vi "player tansition data for all.vi"() -> ()   [LabVIEW 2013]
panel:
  in  "DU opp ALL":string[](array[string])=["0 3 0 1 0 -3 0 -3 3 0\r\n", "1 -4\r\n", "2 0 2 0 -1 0 -3\r\n", "0 4\r\n", "0 -1 2 -1 0 2 0 3 0 1 -4 1 0 -4 4 -4\r\n", "0 -1 0 -4 0 -2 0\r\n", "1 -1 1 0 -4\r\n", "-1 0 -4 0 1 0\r\n", "0 3\r\n", "-1 1 0 -4 1 0 -4 0 -1 2 0\r\n", "1 0 -1 0 2\r\n", "0 -1 -4 1 0 -3 3\r\n", "2 -1 0\r\n", "0 4 0 2 0 -3 0 1 -1 0 1 -4 4 -4 4 -4 0 3\r\n", "0 -4 4 -4 0 -1 2 0 3 -3 0 -3 3 0 -4 1 0 -3 0 3 -2\r\n", "0 3 0\r\n", "0 4 0 1 0 -4 4\r\n", "0 -1 0 4 0\r\n", "1 -1 0 4 0 2 -2 0 -4 1 -4 4 -3 0 -4 0 -3 3 0 -4 1 -1 2 -1 0 4\r\n", "0 3 0 4 -4 4 -4 1 -4 1 -4 4 -4 1 -4 0 -3 3\r\n", "", "0\r\n", "0 4 -4 0 -4 0 4 -4 0\r\n", "1 -4\r\n", "0 4\r\n", "0 1 -4 1 -4 0 -4 4 -4 0\r\n", "-2 2 0 -3 3 -3 0 3 0\r\n", "1 0 4 0\r\n", "0 3 0 1 0\r\n", "0 4 -4 0 -4 1 -4 0\r\n", "0\r\n", "0 -4 4 -4 0 -3 3 -2 0 2\r\n", "0 3 0 1 0 -4 4 0 -3 3 0 -4 0\r\n", "0 1 0 3 -2 3\r\n", "0 2 -2 3 -3 0 -3 3 -2 2 0 -4 4 -4 1 0 4 0 2 -2 0 4 0 4 0 2 -2 2\r\n", "0 -3 3 0 -2\r\n", "1 0 -2 0 4 0 1 0 -2 2 -2\r\n", "-2 0 3 0\r\n", "-4 0 -2 0 3 -3 0 -2 2 -2 0 -4 0 3 -2 0\r\n", "0 -3 4 0 1 0 -2\r\n", "-2\r\n", "-4 0\r\n", "-2 0 -3 4 -3 4 -4\r\n", "0 1 -4 0 -2 2 -2 0 -4 0 -3 3 -2 3 0 1 0\r\n", "0 3\r\n", "0 2 0 3 0 1 0 -2 2 -2 3 0\r\n", "-1 0 -1 1 0 4 -4 4 -4\r\n", "0 -3 4 -3 -2 2 -2 3 -2 2 -2 0\r\n", "2 0 -3 3\r\n", "0 3 0 -1 0\r\n", "0 3\r\n", "0 3 0 3\r\n", "-4 0 -4 1 -4\r\n", "2 -2 0 3 -3 0 1 0 -1 0 4 -3 0 2 -2 0\r\n", "0 1 0 4 -4 4 0\r\n", "0 1 0 -3 3 -3 0\r\n", "0 -3 4 0 -4 1 0 -2\r\n", "0 3 0 -2\r\n", "2 0 -3 3 -2 2 0 -2 0 -3 4 -3\r\n", "0 1 0 3 0\r\n", "0 3 0 -2\r\n", "-4 0 3 0 2 -1 0 3 0\r\n", "2 0 4 0 -2 2\r\n", "0 -3 4 -3 0 -2 2 -2 0 4\r\n", "0 3 -2 0 -3 4 0 3 0 1 -1 0 -1 0\r\n", "0 -3 4 -3 0\r\n", "2 0 3 -3 0 -4 0 -2\r\n", "-1 0 3 -3 0 1 0 4\r\n", "0 1 0\r\n", "0 -1 0 -1 1 -1 0\r\n", "0 -3 3 -3 0 1 -4 0 -1 0\r\n", "2 0 3 -2 0 -2 3 -2 0\r\n", "0 1 0\r\n", "2 0\r\n", "0 1 -4 0 -4 0 -3 4 -4 0 2 0 2\r\n", "0 3 -2 2 0 -4 0 -3 0 1 -4 4 0 2 0 -3 3 -3 0 -2 2 0\r\n", "0 2 0 3 -3 0 3 -3 0 1 0 4 -3 0 2 0 -2 0 4 -4 1 -1\r\n", "-4 1 0\r\n", "0 2 0\r\n", "0 1 0 -4 0 -4 0 -1 0\r\n", "0 4 -4 0 -4 4 -3 0 2 0 -1 1 -1 0 3\r\n", "0 2 0 -4\r\n", "0 3 -2 0 -2 0 -2 3 -2 2 -2 3\r\n", "0\r\n", "0 -3 4 0\r\n", "0 2 0\r\n", "0 -3 4 -3 0 -2 2\r\n", "0\r\n", "0 2 0 1 0 -3 4\r\n", "2 0 -4 1 0 3 0 -4 1 -1 0 4 -4 1 0 2 -2\r\n", "1\r\n", "2 0 -1 0 -1\r\n", "1 0 4 -4 0 2 0 -1 0 -1 0 4 -4 0 2 0 3 -2 3 0 -1 1 0 4\r\n", "0 1 0 -2 0 -1 1 -4 4 0 -4 0\r\n", "0 -1 0 -1 0\r\n", "2 0 -1 1 0 4 -4 1 0 1 0 -3 0 -2 0 -4 0 4 0 1 0\r\n", "0 4 -4 1 -4 1 -4 0 -1 0 -1 0 -1 1 0 -4 4 0 -1 0\r\n", "0 3 -2 0 3 0 2 0 2 0 -4 1 0 -3 0 1 0 4 -4 0 3 -3 0 1 0 -1 0 -1 -4 4 0 2\r\n", "1 -4 1 -1 0 -4 1\r\n", "2 -1 0 -4 1 0\r\n", "1\r\n", "2 0 1 0 -4 1 -4 4\r\n", "0 2 0 -2 2 -1 0 4 -4 0 -4 4\r\n", "1 0\r\n", "2 0 -4 4 0 2 -1 0 -4 4 0 1 -1 0 4 0 2\r\n", "0 4 -4 1 -4 0 -4 1 -4 4 -4 0 1 -1\r\n", "0 -1 1 0 -4 0 -1 0 3 -2\r\n", "1 -4 1 0 1 -4 4 -4 1 0 1 -4 1 0 4 0 4 -4 0 4 -4 1 0 4\r\n", "2 0\r\n", "1 0 1 0 -3 0 -3 3 -2 2 -1 0 -1 0 -1 0 -4 1 0 2 -2 2 0 4 -3 0 4 -4 1 0 4 0 -1 2 0 -3 0 3 0 1\r\n", "2 0 2 0 -4 4 -4 0 -4 4 -3 0 2\r\n", "0 3 0 2 -1\r\n", "0 4 0 -2 0 3\r\n", "0 4 -4 1 0 -4 0 4 -4 0 2 0 -1 1 -1 0 -1\r\n", "1 0 4 -4 1 0 4 -4 0\r\n", "2 -1 0 -1 0 4\r\n", "1 -4 1 0 4 0 2 0 2 0 -3 0\r\n", "2 -1 0 -3 0\r\n", "0 -1 1 0 1 -4 4 -4 0 -1 0 -3 3 0 1 0\r\n", "0 2 0 3 0\r\n", "1 0 1 -4 1 0\r\n", "2 0 3 0 3\r\n", "0 3 0\r\n", "0 2 0 3 0 3 0 3 -2 0 1 -4 1 -4 4 -4 1 -4 4 -4 4 -4 1 -4 0 -2 0 1 0 -4 4 -4 0\r\n", "0 4 0 -2 0 1 -4 4 -4 1\r\n", "0 4 -4 1 -4 1 0 1 -4 1 -4 1 -4 0 2 0 3 0 2 0 -3 3 0 3 -2 0 -1 1\r\n", "1 0 1 -4 1 0 -1 0 -4 0 -1 0 4 0 4\r\n", "0 1 0 1 0 1 -4 1 -4 4 0 -1 0 3 0 -1 0 4 0 2 0 2 0 4 -4 4\r\n", "0 2 0 1 0 -4 1 0 4\r\n", "2 0 -1 0 2 0 4 0 -2 0 3 0 2 0 2 -2 2\r\n", "0\r\n", "0 2 0 -2 0 -1 1 -1 0 -4 1 -4 1 -4 1 0 -4 4 0 -4 0\r\n", "1 0 -1 0 1 -4 1\r\n", "2 -1\r\n", "0 1 0 3 0 1 0 4 0 4 -4 1\r\n", "0 4 0 2 0 1 0 1 0\r\n", "-4 1 0 -4 0 -2 0 2 -1 0 4 -4 1 0 4 -4 0 2 0\r\n", "0 -3 3 0 1 0 1 0 -4 4 -4 0 1 0 4 -4\r\n", "2 0 1 0 1 0 2 0 3 -2 3\r\n", "0 4 0 2 0 -2 2 0 -4 4 -4 0 3 0 4 0 2 -1 0 4 -4 0 -4 4 0 2 0 -2 3 -2 2 -1 0 -4 4 -4 0 2 0 -3 0 -3 3 0 4 -4 0 2 -1 1 -4 4 0 2\r\n", "1 0 -4 1 -4 0 -4 4 0 -1 0 -4 1 0 1 -4 1 -4 1 -1 0 4 -4 0 3 0 -1\r\n", "0 -3 3\r\n", "0 1 0 -3 4 -3 0 2 -2 0 -2 0 -3 4 -3 0 -2 2 -2 0 -3 4 0 2 0\r\n", "-4 0 -4 4\r\n", "0 4\r\n", "0 2 0\r\n", "-4 0\r\n", "0 -3 0\r\n", "-2 2 0 -3 3 0 3 -3 0 -2 2 -2 3 -3 3 -2 0 -3 4 0 4\r\n", "0 -3 3 0 2 0 -4 1 0\r\n", "-4 1 -4 4 0 1 -1 0 3\r\n", "0 -3 4 0 -3 3 -3 0 -2 0 -4 0 -2 0 -3 3 0 1 0 -4 4 0 -3 3 0 3\r\n", "0 4 0 -4 0 -1 0 1 -4 4 -4 0\r\n", "0 1 0 -3 4 0 2\r\n", "0 2 0 3 -3 -4 1 -4 4 -3 4 0 -4 0 -3 4 -3 0 -2 2 0 -4 0 3 -2 3 -2 0 -3 3 0\r\n", "-4 1 0 -4 0 3 -2 0 -3 4 0 2 0 3 -3 0 1 -4 0 2 -2 0 -2 0 -3 3 0 3\r\n", "0 -2 2 -2 0 -2 2 0 3\r\n", "0 -3 3 0 3\r\n", "0 2 0 4 0 2 -2 0 -3 4 0 1 -4 0 -2 2 0 -4 1 0\r\n", "0 -3 3 -3 0 1 0 3\r\n", "0\r\n", "0\r\n", "0 4 0 -2 0 -3 4 -3 0\r\n", "0 1 -4 0 -4 0 2 -2 3 0 2 0 1\r\n", "0 3 0\r\n", "0 -3 3 -3 0 3\r\n", "0 3 0 4 -4 0 -3 3 -3 0 2 0 2 0 4\r\n", "0 4\r\n", "0 2 0 -4 0 1 0 1 -4 0 4 0\r\n", "0 2 -2 0 3\r\n", "-4\r\n", "2 0 1 -4 0 4\r\n", "0 4 0\r\n", "2\r\n", "0 1 -4 0 4 -3 0 -4\r\n", "0 2 0 3\r\n", "0 2 0 -3 3\r\n", "0 2 0 -2 2 -2 0 -3 4 -4 1 0 -3 4 0\r\n", "0 -4 0 -4 1 0 2 0 2 0 3 -3 0 -4 1 0 3 -2 2 0 -3 4 -3 0 3 0 3\r\n"]
  in  "CL opp ALL":string[](array[string])=["0 3 -2 0 -2 0 -2 0 -2 2 -2 0 3 -3 0 2 0 -3 4 -3 0\r\n", "0\r\n", "0 3 -3 0\r\n", "0 2 -2 0 3 -3 0 1 -4 -1 1 0 -4 0 3 0\r\n", "-4 1 0 2 -1 0 3 -3 0 -4 0 2 0 3 0 -4 1\r\n", "0 2 0\r\n", "0 3 -2 0 3 -3 0 3 0 2 0 3 0 3 0 -2 2 -2 0 -2 3\r\n", "-4 1 0 -2 3 0 -1 0 3 0\r\n", "0 1 -4 0 -4 0 3 0 2 -2 0 4 -4 1 0 3 -3 0 -2 3 0 -4 0 2 0 -4 0\r\n", "0 -4 4 -3 0 3\r\n", "0 3 -2 3\r\n", "0\r\n", "0 -3 3 -3 0 2 0 3 0 -2 2\r\n", "-4 1 0 3 0 -3 -2 3 0 1 -4 0 3 -3 0 1 0 -2 0 2 0\r\n", "-1 0 -2 3 -2 0\r\n", "0 3 0 3 -3 0 -4 0 -3 3 -3 0 -4 0 4 -3 0 1 -4\r\n", "-4 0 -2 0 3 -3 0 -3 3 0 -4 0 2 0 -4 0 2 -2 0 -3\r\n", "0 3 0 -3 4 0 2 0 3 -3 0 -4\r\n", "0 3 -2 0 4 0 -2 0 3 -3 0 3 0 3 -3 0 -2 0 4 -3 0\r\n", "0 4 0\r\n", "0 2 0 -4 0 -4 0 3 -2 0 -3 3 0 2 -2 3 -3 0 -4 1 0 -4 0 -2 0 4 0 -2 0 -2 0 1 0 4 0 -2 2 -2 0 3\r\n", "0 4 0 -2 2 0 3 0 -4 1 -4 0\r\n", "-4 0 -4 0 -4 0 -3\r\n", "0 4 -4 1 -4\r\n", "-4 0 -2 3 -2 3 0 -4 4 -4 4 -4 0 4\r\n", "0 3 0 -2 0 1 0 4\r\n", "0 3 0 2 0\r\n", "0 3 0 -4 0 3 -3 0 -4 1 0 4\r\n", "0 4 -4 4 -4 0 -1 0\r\n", "-2 0 3 0 -4 0 -2 2 0 3 -3 0 -2 2 -2 -3 3 -3\r\n", "-4 0 -3 0 3 -2 0 3 -2 2 -1 0\r\n", "0 3 -3 0 1 -4 0\r\n", "0 2 0\r\n", "0\r\n", "-4 0 4 0 -4 0 -4 4 0 2 0 4 -3 0 2 -2 0 -2 3 0 -2 2 -2 0 -2 0 -2 3 -3 0 4 0 4 -4 1 0 -3 3 0 -4\r\n", "0 -2 3 0 -4 1 -4 0 -2 2 -2 0 -2 3 -3\r\n", "-4 0 -2 3 0 2 -2 3 0 3 -3 0 -3 3 -3 0 3 -3 4 0 2 0 4 0 -4 0\r\n", "0 3 0 3 0 -1 2 0 3 -3\r\n", "0 3 -3 0 2 0 3 -3 0 -3 3 -2 0 1 0 1 0\r\n", "-4 0 -3 3 -2 2 -2 0 3 -3 0 -2 2 0\r\n", "0 3 -3 0 -4 1 0 4 0 -3 3 -3 0 -4 1 -4 0\r\n", "0 2 0\r\n", "-4 0 4 -4 4 -4 0 4 0 2 0 3 0 3 -2 2 0\r\n", "0 3 -2 0 3 0 -2 2 0\r\n", "0\r\n", "0 3 -3 0 -4 0 -4 0 -2 0\r\n", "-4 0 -4 0 -3 3 0 3 -3 0 -4 1 0\r\n", "0 3 0 -3 4 -4 1 -4 0 -3 3 -3 0 -2 2 0 1 0 -2 0 -4 1\r\n", "0 2 -2 3 -3 0 4 -4 4 0 2 0 3 -3 0 -2 0 1 0\r\n", "0 3 -2 0 3 -3 0 1 -4 1 0\r\n", "-4 0 -4 0 3 0 3 0 3 0 2 0 -2 0 -2 0 -3 3 -3 0 1 0 3 -3 0 -2 0 4 0 -4 0 -2 3 0 -4 1 -4 1 0 4 0 -2 2 0 -4 0 3 0 -4\r\n", "0 3 0 3 0 -2 0 3 -3 0 3 0 2 0 -3 4 -4 1 0 3 -3 0 1 0\r\n", "0 2 0\r\n", "0 -1 0 4 0 -1 0 1 -4 4 -4 1 0 -4 1 -4 0 1 0 4 -4 0\r\n", "0 -2 0 2 0\r\n", "1 -1 0\r\n", "0\r\n", "-1 0 3 0 4\r\n", "0 2 0 4\r\n", "0 -1 0 -4 0 1 -4 1 0 -4 1 0 3 0\r\n", "1 -1 0 -4 0 -3 4 0 -1 0 3 -2 2 0 -3 0\r\n", "0 -1 0 2 0 3 0 2 0 4 0\r\n", "0 3 0 1 -1 0 -1 2 -1 0 1 -4 1 0 2 0 3 0 -4 0 2 0 1 0 2 0 -2 0 1\r\n", "2 0 -2 3 0 -1 0 -1 0 -1 0 3 0 2 0 4\r\n", "0 3 -2 0 1 0 -1 0\r\n", "0 -4 4 0 2 -1 0 1 0 1 0 3 0 4 0 -4 4 -4 0 -4 0 -1 2 -1 0 1 -4 1 0 -2 0\r\n", "0 3 0 3 -2 0 -4 0 -4 0 3 0 1 0 -2 3 0 -4 4 -4 0 2 0 3 0 -4 4 -4 0 2 0 4 -4 0\r\n", "1 -4 1 -4 4 -4 1 -4 1 -4 0 -3 3 0\r\n", "2 -1 0 4 -4\r\n", "1 0 3 0 2 0 -4 1 0 -2 0 -2 3 0 1 -4 1 0 3 -2 2 -1 0 -3 4\r\n", "0 3 -2 0 -1 0 3 0 -2 0 -4 4 0\r\n", "-1 0\r\n", "-1 0 -2 0\r\n", "1 -1 0 3 0 1 0 1\r\n", "2 0 2 0 -2 3 -2 0 -1 0 3 0 1 0 3 -2 -1 0 4 0 2 -1 1\r\n", "1 0 -2\r\n", "2 -1 0 -1 0 4 0\r\n", "0 3 0 1 -4 0 -1 0 3 -2 0 1 -4 1 0 1 0 3 0 -4 1 0 3 0\r\n", "-1 0 3 0 3 0\r\n", "1 -1 0 3 -2 0 -1 0 -1 0 3 -2 2 0 3 0 2 -2 0 3 0 -2 0\r\n", "0 3 0 4 -4 1 -4 1 0\r\n", "0 -1 0\r\n", "0 3 0 4 -4 0 3 0\r\n", "-1 0 3 -2 0 1 0\r\n", "0\r\n", "-1 0 4 0 2 0 -2 3\r\n", "2 -1 0 4 -4 0 -1 0\r\n", "-4 1 0 -1 0 -1 0 -4 4 -4 0 -1 0 -4\r\n", "2 -1 0 3 -2 0 1 -4 1 0 -2 0 1 -1 0 -2\r\n", "0 3 -2 2 0 3 -3 0 1 -4 1 0 -2 0 4 0 -4 1 -4 0 3 0 1 0 4 -4 0 -4 4 -4\r\n", "0 -1 0\r\n", "0 3 0 4 0\r\n", "0 2 0 -1 0 3 0 -1 0 -1 0 1 0 1\r\n", "0 -1 0 -2 -1 1 0 -3 0 3 0 2 -1 0 3 0 1 -4 4 0 4 -4 1 -4 4\r\n", "0 3 0 3 0 4 0 2 -2 0 4 -4 0 2 0 1 -4 4 -4 0 3 0\r\n", "0 -1 0 4\r\n", "1 0\r\n", "2 0 4 -4 0 1\r\n", "-4 1 -1 0 2 0 1 -4 0 -3 0 2 -2 0 4 0\r\n", "0 -1 0 3 0\r\n", "0 3 0 1 0 1\r\n", "0 -1 0 4 -4\r\n", "1 -1 0\r\n", "0 3 0 4\r\n", "2 0 -2 3 -2 0 4 0 -4 1 -4\r\n", "0 -1 0 3 -2\r\n", "0 -3 3 0\r\n", "0 3 0 -2 0 4 0 2 -2 0 4 0 4 -4 1 -4 0\r\n", "2 0 -3 3 0 -2 0 1\r\n", "0 3 0\r\n", "-4 0 2 0 3 -3 0 -3 4 0 -4 1\r\n", "-2 2 0 1 -1\r\n", "0 -1 0 4 -4 1 -4 1\r\n", "-4\r\n", "-2 2 0 3 0 -4 0 -3 3\r\n", "-4 1 0 4 -4 1 -4\r\n", "0 4 -4 0 4\r\n", "0 4 0 -4 0 1 -4 0 -4 4\r\n", "0 1 -4 0 -4 0 -2\r\n", "-2 2 0 -4 1 0 -4 0 4 0 3 0 -1 1 -1 1 0 -3 0 -2 2 0 -4 4 -4 0 2\r\n", "0 -3 3 -3 0\r\n", "-4 0 -1 2 0 -3 4 0 2 -2 0 3 -3 0 1 -4 0 -4 0 -4 0 -3 3 0 -3 4 0 2\r\n", "-2 0 3 0 -2 2 -2 0 -2 0\r\n", "-4 0 3 0 -4 1 0 -3 4\r\n", "-2 2 0 2 0 -2 0 -3 3 0 -4 1 0\r\n", "-4 0\r\n", "0 -3 3 0 2 0 -3 4 0 -2 0 1 -4 0\r\n", "0 2 0 3\r\n", "0 4 -4 1 -1 2 0 -3 0 1\r\n", "0 -2 0 -3 4 0 1 -4 0 -3 3 0 -4 0 4 0 2 -2 0 -2 0 -4\r\n", "0 3 -2 0 4 0 4 0 -1 0 -3 3 0 1 -4 0 -4 0 4 0 2 -2 0\r\n", "-2 3 -2 0 1 -4\r\n", "-4 0 -1 0 -3 3\r\n", "0 4\r\n", "0 3 0 -3 3 -3 0 -1 0 2 -2\r\n", "-2\r\n", "-4 0 -2 0 2 0 1 0 -4 0 4 0 2 0 -3 4 0 2 0 -2 0\r\n", "0 2\r\n", "-2 0\r\n", "-4 0 3 0 -4 1 -4 0 -4 4 -4 4\r\n", "0 1 -4 0 -3 3 0 1 -4 0\r\n", "-2\r\n", "-2 2 0 2 -1 0 4 0\r\n", "1 -4 1 0 -4 0 3 0 -1 0 -4 0 2 -2 0 4 0 2 0 4 -4 0 2 -2 0 1 0 -4 1 0 4 -4 0 1 -4 1 0 4 -4 0 2 0 4\r\n", "-2 2 0 -1 0\r\n", "0 -1 0 -1\r\n", "4 1 -1 0 4 -4 0 -1 0\r\n", "0 -2 2 0 -2 2 -2 0 4 -4 0 -1 0 -1\r\n", "0 -4 4 -4 -1 0 -1 0 1 -4 4\r\n", "-4 1 0 -1 0 -1 0 4 -4\r\n", "2 -1 0 1 0 4 -4 0 2\r\n", "0 1 0 4 -1 4 -4 1\r\n", "0 -1 0 4 0 -1 0 -1 0 2 -2\r\n", "-4 1 -4 1 0 1 0 -1 0 4 -4 0 2 0 3 -2 0 1 0 1 0 -1 2 -1 0\r\n", "-2 2 0 -1 2 -1 0 -3 3 0 -1 0 4 0 1 -4 0 -4 0 4 0 2 0\r\n", "1 0\r\n", "-2 2 -2 2 0 -3 0 1 -4 1 0 1 -4 1 -4 0 -3 3 0 4 0 1 -4 4 0\r\n", "1 -4 1 0 -4 1 0 -4 1\r\n", "0 -1 2 -2 2 0\r\n", "2 0\r\n", "-4 1 -4 1 0 -3 0 -1 0 1 -4 1 0 -1 1 -1 0 1 0 1 0 4 -1 4\r\n", "0 -4 0 1 -4 0 1 0 1 0 -3 3 0 2 -2 2\r\n", "-2 2 0 -1 0 -3 4 0\r\n", "0 1 -1 0 4 -4 1\r\n", "1 -4 1 0 4 -4 1\r\n", "0 4 -4 0 -1 0 -2 0 -1 0 -1 0 -3 3 0 -1 0 -1 0 -1 0 2 0 4 -4 1\r\n", "-2 2 0 2 -1 0 4 -4 0 -4 4 -4 -1 -4 1 0 -4 4 -4 0 2 -2 3 0 1 0\r\n", "1 -4 1 -4 0 -3 0 3\r\n", "0 -1 0 1\r\n", "0 -1 0 -1 0 -3 4 0 -4 0 -1 2 -1 0\r\n", "0 2 0\r\n", "1 -4 1 0\r\n", "2 0 4\r\n", "0 -1 0 -3 -1 -3 0 1 -4 0 -4 0 -3 0 1 -4 0 3 -2 -1 0 -4 1 0 -4 0 4 -4 0 2\r\n", "0 -1 0 1 0 -1 2 -1 0 -2 0 4\r\n", "0 -1 0 1\r\n", "0 1 -4 1 0 -1 0 -3 -1 -3\r\n", "0 -1 1\r\n", "0 -1 0 3 0 1 -4 1 0 4 0 -4 1 0\r\n"]
  in  "CJ opp left":string[](array[string])=["-2 2 -1 0 1 -4 0 3 -2\r\n", "1 -1 0 4 0 2 -2 3 0 1 -4 1 0 -3 4 0 3 0 4 0 4 0 -4 0\r\n", "-1 0 4 -4\r\n", "-1 0 -1 2 0 2 0\r\n", "-1 0 3 -2 0 2 -2 3 -2 2 -2 0 -3 4 0 1\r\n", "-2 2 -1 0 2 0 3 -1 3 -2 2 0 -2 2 -2 0 1 0 2 0\r\n", "1 -4 1 0 4 -4 0 2 0\r\n", "2 -2 0\r\n", "0 4 -4 -1 0 -1 1 -1 0 4 0 -2 3 -2 0\r\n", "-1 0 2 -1 0 4 -4 0 -4 0 4 0\r\n", "0 -3 0\r\n", "1 0 -1 2 -1 0 3 0 3 -2 3 -2 0 2\r\n", "2 0 2 0 -2 3 -2 2 -1 0 4 0 2\r\n", "-1 1 -4 1 0 1 0 -4 4 -4 0 3 -2 2 -1 0 3 0 -1 1\r\n", "2 0 -1 1 -1 0 3 -2 3 0 2 0 3 -2 0 -4 0 4 -4 0 4 0\r\n", "0 -1 0 3 0 2 -2\r\n", "1 -4 1 -1 0 2 0 3 -2 3 -2 3\r\n", "2 0\r\n", "-1 0 3 0 3\r\n", "1 -4 1 0 -4 4 -4 0\r\n", "-2 2 -1 0\r\n", "0 1 0 4 0 3 0 -2 0 3 0 4 0 2 -2 0\r\n", "0 3 -2 0 4 0 -2 2 -2 0 -2 0 4 0 -2 0 2\r\n", "2 0 1 -1 0\r\n", "1 0 -3 4 -3 0 -2 0 3 0\r\n", "0 3 -2 0 4 0 -3 3 0 3 -2 0\r\n", "2 0 3 0 1 0 3\r\n", "1 0 3 -3 0 4 -3 0\r\n", "-2 2 -2 0\r\n", "0 1 0 -3 4 0 3 -2 3 0 1 0 4 0 -1\r\n", "0 3\r\n", "-2 2 0 3 0 -2 0 2 0 -2 0 3 0 -4 0 -2\r\n", "0 3 0 -3 4\r\n", "0 3 -2 2 -2 3 -2 0\r\n", "-1 0 3 0 3\r\n", "2 0\r\n", "0 -3 0 1\r\n", "1 0 4 -4 1\r\n", "-2 2 0 4 0 -2 0 -2\r\n", "1 0 4 0 1 0 -3 3\r\n", "-2 2 0 3 -2\r\n", "1 0 -3 4 -3 0 3 0 3 0 -2 0 3 -2 0 1 -4 0 3 0 -2 0 3 -3 0\r\n", "-2 2 0 2 0 3\r\n", "0 3 -2 0 3 0 -4 1\r\n", "0 1 0 -4 4 0 -2 0 3 0 -4 0 4 0 -4 1 0 3 -2 3 0 -1 1 -1\r\n", "2 0 -3 4 -3 0 2 0\r\n", "0 3\r\n", "0 3\r\n", "-1 0 4\r\n", "0 3\r\n", "-2 3 0 1 -4 0 -2 2 -2 3 0 4\r\n", "2 -2 0 4 0 -4 1 -4 0 3 -2\r\n", "1 0 2\r\n", "0 3 0 2 -2 3 -3 0 1 0 -3 3 0 4 0 2 -2 2 -2 3 0\r\n", "2 0 -2 3 2\r\n", "0 1 0 4 -4 1 -1 2 -2 3 -3 0 -2\r\n", "0 -3 4 -3 0 2\r\n", "0 2 -2 3\r\n", "0 -4 0 -4 1 0 3 0 1 0 2 -2 0 -3 4 0 4 -3 0 3 -3 -2 0 -3 4 0 -4 0 3 0\r\n", "-2 2 -2 3 -3 0 -4 1\r\n", "0 -2 0 2 0 4 0\r\n", "0 -3 0 -4 0 -3 4 0 -2 3 -3\r\n", "2 0 -2 2 0 4 0 1 0 -2 3\r\n", "0 4 0 3 -2 3 0 -4 4 0 4 0 3 0 3\r\n", "2 0 -2 0 4 0 3 -2 2 -2 3 0 -2\r\n", "1 0 3 -3 0 3 0 3 -2 3 -2 3 0 3 0 -1 0 4 0 -4 1 0 3\r\n", "2 -2 0 -3 4 -3\r\n", "0 1 0 3 0 -2 2 -2\r\n", "1 0\r\n", "2 0 -2 3 -2 2 0\r\n", "1 0 -4 4 0 3 -2 3 -2 0 4 -3 0 -3 4 0 -4 1 -4 0 2 -2 0 3 -3 0 1 0 3 0 -2 3 0 4 0 -4 1 0 3 0 -3 4 0 2\r\n", "0 -3 4 -3 0 1 0\r\n", "0 3 0 4 0 -4 1 0 -2 0\r\n", "2 -2 0 -2 0 -4\r\n", "-1 0\r\n", "2 0 4\r\n", "1 0 3 0\r\n", "2 0 -4 4 0 1 0 3 -2 0 4 0 -4 0 3 0 -2 3\r\n", "0 2 -2 0 -4 0 -4 4 -3 0 -4 1 0 4 0 -3 3 0\r\n", "1 0 4 -3 0 2 -2 0 4 0 -3 4 -3 0 -4 0 -3 0 -4 1 0 -2 3 -2 0 1\r\n", "2 -2 3 0\r\n", "2 -1 0 4 0 1 0 3 -2\r\n", "0 3 0 -2 3 -2 0 -2 3 -2 2 -1 0 3 0\r\n", "1 0 1 0 4 -4 0 3 0 3 -2 0 4 0 3 -2\r\n", "0 3 -2 0 -1 1 0 2 -2 2 0 -3 4\r\n", "2 0 4\r\n", "0 -4 4 -4 0 1 -1 0 4\r\n", "-1 0 4 -4 0 -4 4 -4 0 2 0 -4 0 -3 3 -2 3 -2 0 -4\r\n", "2 0 -1 2 -1 0 1 -1 0 3 0 -2 0 3 0 -3 0 -3 0 -4 4 -4 1 -1 2 -1 1 0 3 0\r\n", "0 3\r\n", "1 0 -3 0 1 -4 0 2 0 -2 3 0 4 -4 0 -1 0 3 0 1\r\n", "0 -1 2 0 -3 4 0 -1 0 4 -4 4 -4 0 2 -1 1 0 -3 3 0\r\n", "0 3 -2 3 0 4 0 1 0 4 0 -4 4 -4 0 -4 4 -4 0 3\r\n", "2 0 3 0 1 0\r\n", "1 0 -4 1 -1 0 -2 -1 3 -2 2 -2 0 -3 0 1 -1\r\n", "2 0 3\r\n", "-4 1 -1 0 3 0 3 0 1\r\n", "0 4 0 -4 1 0 1 0 3 0 4 -4 0 -4 4 0\r\n", "2 0 -4 4 0 -1\r\n", "0 3 -2 2\r\n", "0 4 0 1 -4 4 -4 0 2 0 -3 4 0 4 -4 0 3 0 -1 1 -4 4 0 1\r\n", "0 1 -1 0 -4 0 4 0 1 0 4 0 2 0 -4 4 0 2 0 3 0 4 -4 0 3 0 4 0 -4 4\r\n", "1 0 -4 4 0 2 -1 0\r\n", "2 0 4 -4 1 -1 0 4 0 -2 2 0 4 -4 0 1 0 4 0 2\r\n", "0 4 0 3 -2 0 4\r\n", "0 3 0 -2 3 0 1 -4\r\n", "1 -4 1 0 -1 0 3 -2 2 0\r\n", "2 0 -1 0 3\r\n", "0 -1 0 2 0 -3 4 -4 0 3 0 1 -1 0 -4 4 -4 0 2 -1 1 0 3 0 4 -4 0 3 0 1 0 3 -2\r\n", "2 -1 0 3 0 4 -4 0 1 -4 1 -1 0 -4 4 0 -4 0 3 -2 0 4 -4 4 -4 0 2 -2 0 1 0 4 0 3 0 3 -2 3 -3 0 3 0 -3 0 1 -4\r\n", "1 -1 0 -2 3 -3 0 -4 0 -3 0 3 -2 0 3 -2 2\r\n", "0 4\r\n", "2 0 -2 3 0 2 -1 0 -3 0 -2 3\r\n", "1 0 3 0 3 0 -2 3 -2 0 -2 3 -2 0 3 0 1 -1 0 3 0 3 0 4 -4 0 1 -1 0 3 0 -3 0 -4 4 -4 0 3 0 -1 1 -4 1\r\n", "0 -1 2 0 3\r\n", "2 0 3 -2 0\r\n"]
  in  "CJ opp Right":string[](array[string])=["-2 0 3 0 -3 0 4 -4 0\r\n", "0 3\r\n", "0 4 -3 0 -4 1 0 4 -3 0\r\n", "0\r\n", "-2 0 3 -3 0 -4 1 -4 0 3 -3 4 -3 0 2 0 3\r\n", "0 3 0 1\r\n", "0 1 0 3\r\n", "0 3 -2 0 4\r\n", "0\r\n", "0 -3 4 0 2 -2 0 -3 0 3 -2 3 -3 4\r\n", "0 -3 4 -3 0\r\n", "-2 0 -2 2 0\r\n", "0 3 -2\r\n", "0 4 -3 0 3 -2 0 -3 4 -3 0 3 -2 2 -2 0 4 0\r\n", "2 0 1 -4 0 3 0 -4 4 0 -4 4 0 2 0 4 0 -3 4 -3 0 -4 0 4\r\n", "0 4\r\n", "-2 0 -2 0 3 0\r\n", "0 3 0 -2 3\r\n", "0 4 0 4 -4 0 2 0 -4 4 -3 0 -2 2 -2 0 4 -3 0 2 0 3 0\r\n", "0 4 -3 0 1 -1 0 3 0 -2 2 -2 0 -3 4 -3 0 4 -4 1 0\r\n", "", "0 -3\r\n", "2 0 3 0 1 0 -2 3\r\n", "0\r\n", "1 -1 0\r\n", "0 -2 3 0\r\n", "0 1 0 4 0 4 -4 4\r\n", "0 1 -1 0 3\r\n", "0 2 -2 3 -3 4\r\n", "-2 2 0 -2 3\r\n", "0 -1\r\n", "0 4 -4 4 0 3 0 -2 0 -4 0 1 -4\r\n", "-2 0 4 0 -3 3 0 -2 2 -2 0 -4 0 4 0\r\n", "0 -1 0 -4 4 -4 1 -4 0\r\n", "1 -4 1 0 2 0 -3 0 2 0 -2 0 1 0 1 -4 4 -4 1 0 3 -2 0 -4 4 -4\r\n", "0 1 -4 4 -4 1\r\n", "0 3 0 -3 3 0 1 0 1 -4 4\r\n", "0 1 -4 0 1 -4\r\n", "0 3 -2 0 1 -4 1 0 2 0 4 0 4 0 -1 2 -1 0\r\n", "1 0 -1 0 2 0 4 -4\r\n", "-4\r\n", "-1 0 4\r\n", "0 1 -1 0 1 -4 0\r\n", "-1 0 1 -4 0 3 0 2 0 4 0 -4 4 -4 0 -1 0 -4 0 -2 0 4\r\n", "0 4 0\r\n", "0 4 -4 0 2 -1 0 2 0 4 -4 1 -4 4 0 3\r\n", "0 4 0 2 0\r\n", "1 0 -1 1 0 -4 1 -4 1 0 -4\r\n", "0 3 -2 0 -4\r\n", "2 -1 0 -4 4 -4 0 2 0 4\r\n", "1 0\r\n", "-1 0 -1 1 0 -4\r\n", "0 3 0\r\n", "0 -4 4 -4 0 -4 0 4 0 2 0 1 -4 4\r\n", "-1 0 1 -4\r\n", "-1 0 2 -1 0 2\r\n", "1 -1 0 4 -4 1\r\n", "-1 0 1 -4 4 -4 0 -4 4\r\n", "0 3 0 3 0 1 -1 0 1\r\n", "-1 0 4 0 4 -4 1 0 -4 0\r\n", "1 0 4\r\n", "0 -1 0 2 -1 0 -2 3 -2 0 -4 4 -4\r\n", "0 3 0\r\n", "2 -1 0 1 -4 4 -4 0 2 0\r\n", "0 4 -4 1 0 1 0 1 -4 0 2 0 4 0 4 -4 1\r\n", "1 -1 0 3 0 3 0 1 0 4\r\n", "0 -4 0 -2 0 -4\r\n", "0 -4 4 -4 0 -2 0 2 0\r\n", "-1 0 4 -4 0\r\n", "1 0 -1 2 0 4\r\n", "0 2 0 -2 0\r\n", "0 1 -4 0 -4 0 3 -2 0 -4 0 -4 4 -4 1\r\n", "0 4 0 4 0 4 0 4 0 -2 3 0 3 0 4 0\r\n", "-4 -1\r\n", "-2 0 1 0 -4 4\r\n", "0 4\r\n", "-2 2 0 -1 -4 1 0 3 0\r\n", "-1 0 -1 2\r\n", "0 -1 1 0 4 0 3 -2 0 -2 3 -2 0 4 0 -2 2\r\n", "2 -1 0 4\r\n", "0 4 0 2 0 -2 0\r\n", "1 -1 0 3 0 -4 4 -4 0\r\n", "2 -1 0 3 -2 0 -3 0 3 0 -3 0\r\n", "0 4 0 4 -4 1 -1 0 -3 0 1 -4 1 0 4 0 -4 0 -4 4 -4 1\r\n", "0 -4 1 0 -4 4\r\n", "0 4 0 -2 2 -2 2 -2 2\r\n", "-2 2 -1 0 4 0 2 0 4 0 2 -2 0 4\r\n", "1 0 -1 0 -1 0 1 -1\r\n", "-2 2 -2 3\r\n", "1 0 -1 0 -1 2 0 2 -2 0 -4 0\r\n", "-2 2 0 3 -2 2\r\n", "0\r\n", "1 -1 0 3\r\n", "0 4 0\r\n", "-2 0 1 -4 0 -3 0\r\n", "1 0 -1 2 -1 1 -4\r\n", "0 4\r\n", "-2 0 -1 1\r\n", "0 3 0 3 0 3 -2\r\n", "-4 0 -4 4\r\n", "0 4 0 -4 0 -4\r\n", "-2 2 0 4 -4 0 2 -2\r\n", "-2 2 -2 0 -1\r\n", "0 4 -3 0\r\n", "0 1 0 -1 1\r\n", "-4 0\r\n", "-2 0 3 0 1 0 3 -2 0 -1 0 4 0 3 0 -3 3 -3\r\n", "0 4 0 -2 0 1 0 -4 4 -3 0 1 0 4 0 -4 1 0 3 -3 0\r\n", "0 -1 2\r\n", "2 0 -3 4 0\r\n", "-4 0 -3 3 -3 0 -3 3 0 -2 3 0\r\n", "0 -1 1 -4 4 -3 0 3 0\r\n", "0 -1 2 0 3 0 1 -4 4 0 2 0\r\n", "2 -2 0 -4 0 -4 4 0 -4\r\n", "1 -1 2 -1\r\n", "2 0 -2 0 4 0 2 0 3 0 -2 0 -4\r\n", "1 -1 0 -1\r\n", "0 1 -4 1\r\n", "0 4 0 -1 1 -1 0\r\n", "0 3\r\n", "-2 0\r\n", "1 -4 0 -2 0 4 0 -4 0 4 -3 0 1 -4 0 1\r\n", "0 -3 3 -2 0 3 0 -2 2\r\n", "1 0\r\n", "2\r\n", "0 -4\r\n", "0 4 0 -4 0 -3 3 -3 0 -2 0 -2 0 4 0 -1 1 0 3 0 -4 1 -4 0 4\r\n", "2 0 -1 1\r\n", "0 2 0 4 0 4 -4 0 -1 2\r\n", "0 3 -2 0 3 -2\r\n", "1 0 -3 3 0 -4\r\n", "0 -3 3 0 -1 0\r\n", "2 -2 0 1\r\n", "-4 1 -4 1 -4 0\r\n", "0 4 0 2 0 -4 1 2 -1 0 4 0 1 0 4 -4 4 0 -4 4 0\r\n", "-2 0 3 0 -2 0\r\n"]
  in  "CJ opp ALL":string[](array[string])=["-2 0 3 0 -3 0 4 -4 0\r\n", "0 3\r\n", "0 4 -3 0 -4 1 0 4 -3 0\r\n", "0\r\n", "-2 0 3 -3 0 -4 1 -4 0 3 -3 4 -3 0 2 0 3\r\n", "0 3 0 1\r\n", "0 1 0 3\r\n", "0 3 -2 0 4\r\n", "0\r\n", "0 -3 4 0 2 -2 0 -3 0 3 -2 3 -3 4\r\n", "0 -3 4 -3 0\r\n", "-2 0 -2 2 0\r\n", "0 3 -2\r\n", "0 4 -3 0 3 -2 0 -3 4 -3 0 3 -2 2 -2 0 4 0\r\n", "2 0 1 -4 0 3 0 -4 4 0 -4 4 0 2 0 4 0 -3 4 -3 0 -4 0 4\r\n", "0 4\r\n", "-2 0 -2 0 3 0\r\n", "0 3 0 -2 3\r\n", "0 4 0 4 -4 0 2 0 -4 4 -3 0 -2 2 -2 0 4 -3 0 2 0 3 0\r\n", "0 4 -3 0 1 -1 0 3 0 -2 2 -2 0 -3 4 -3 0 4 -4 1 0\r\n", "", "0 -3\r\n", "2 0 3 0 1 0 -2 3\r\n", "0\r\n", "1 -1 0\r\n", "0 -2 3 0\r\n", "0 1 0 4 0 4 -4 4\r\n", "0 1 -1 0 3\r\n", "0 2 -2 3 -3 4\r\n", "-2 2 0 -2 3\r\n", "0 -1\r\n", "0 4 -4 4 0 3 0 -2 0 -4 0 1 -4\r\n", "-2 0 4 0 -3 3 0 -2 2 -2 0 -4 0 4 0\r\n", "0 -1 0 -4 4 -4 1 -4 0\r\n", "1 -4 1 0 2 0 -3 0 2 0 -2 0 1 0 1 -4 4 -4 1 0 3 -2 0 -4 4 -4\r\n", "0 1 -4 4 -4 1\r\n", "0 3 0 -3 3 0 1 0 1 -4 4\r\n", "0 1 -4 0 1 -4\r\n", "0 3 -2 0 1 -4 1 0 2 0 4 0 4 0 -1 2 -1 0\r\n", "1 0 -1 0 2 0 4 -4\r\n", "-4\r\n", "-1 0 4\r\n", "0 1 -1 0 1 -4 0\r\n", "-1 0 1 -4 0 3 0 2 0 4 0 -4 4 -4 0 -1 0 -4 0 -2 0 4\r\n", "0 4 0\r\n", "0 4 -4 0 2 -1 0 2 0 4 -4 1 -4 4 0 3\r\n", "0 4 0 2 0\r\n", "1 0 -1 1 0 -4 1 -4 1 0 -4\r\n", "0 3 -2 0 -4\r\n", "2 -1 0 -4 4 -4 0 2 0 4\r\n", "1 0\r\n", "-1 0 -1 1 0 -4\r\n", "0 3 0\r\n", "0 -4 4 -4 0 -4 0 4 0 2 0 1 -4 4\r\n", "-1 0 1 -4\r\n", "-1 0 2 -1 0 2\r\n", "1 -1 0 4 -4 1\r\n", "-1 0 1 -4 4 -4 0 -4 4\r\n", "0 3 0 3 0 1 -1 0 1\r\n", "-1 0 4 0 4 -4 1 0 -4 0\r\n", "1 0 4\r\n", "0 -1 0 2 -1 0 -2 3 -2 0 -4 4 -4\r\n", "0 3 0\r\n", "2 -1 0 1 -4 4 -4 0 2 0\r\n", "0 4 -4 1 0 1 0 1 -4 0 2 0 4 0 4 -4 1\r\n", "1 -1 0 3 0 3 0 1 0 4\r\n", "0 -4 0 -2 0 -4\r\n", "0 -4 4 -4 0 -2 0 2 0\r\n", "-1 0 4 -4 0\r\n", "1 0 -1 2 0 4\r\n", "0 2 0 -2 0\r\n", "0 1 -4 0 -4 0 3 -2 0 -4 0 -4 4 -4 1\r\n", "0 4 0 4 0 4 0 4 0 -2 3 0 3 0 4 0\r\n", "-4 -1\r\n", "-2 0 1 0 -4 4\r\n", "0 4\r\n", "-2 2 0 -1 -4 1 0 3 0\r\n", "-1 0 -1 2\r\n", "0 -1 1 0 4 0 3 -2 0 -2 3 -2 0 4 0 -2 2\r\n", "2 -1 0 4\r\n", "0 4 0 2 0 -2 0\r\n", "1 -1 0 3 0 -4 4 -4 0\r\n", "2 -1 0 3 -2 0 -3 0 3 0 -3 0\r\n", "0 4 0 4 -4 1 -1 0 -3 0 1 -4 1 0 4 0 -4 0 -4 4 -4 1\r\n", "0 -4 1 0 -4 4\r\n", "0 4 0 -2 2 -2 2 -2 2\r\n", "-2 2 -1 0 4 0 2 0 4 0 2 -2 0 4\r\n", "1 0 -1 0 -1 0 1 -1\r\n", "-2 2 -2 3\r\n", "1 0 -1 0 -1 2 0 2 -2 0 -4 0\r\n", "-2 2 0 3 -2 2\r\n", "0\r\n", "1 -1 0 3\r\n", "0 4 0\r\n", "-2 0 1 -4 0 -3 0\r\n", "1 0 -1 2 -1 1 -4\r\n", "0 4\r\n", "-2 0 -1 1\r\n", "0 3 0 3 0 3 -2\r\n", "-4 0 -4 4\r\n", "0 4 0 -4 0 -4\r\n", "-2 2 0 4 -4 0 2 -2\r\n", "-2 2 -2 0 -1\r\n", "0 4 -3 0\r\n", "0 1 0 -1 1\r\n", "-4 0\r\n", "-2 0 3 0 1 0 3 -2 0 -1 0 4 0 3 0 -3 3 -3\r\n", "0 4 0 -2 0 1 0 -4 4 -3 0 1 0 4 0 -4 1 0 3 -3 0\r\n", "0 -1 2\r\n", "2 0 -3 4 0\r\n", "-4 0 -3 3 -3 0 -3 3 0 -2 3 0\r\n", "0 -1 1 -4 4 -3 0 3 0\r\n", "0 -1 2 0 3 0 1 -4 4 0 2 0\r\n", "2 -2 0 -4 0 -4 4 0 -4\r\n", "1 -1 2 -1\r\n", "2 0 -2 0 4 0 2 0 3 0 -2 0 -4\r\n", "1 -1 0 -1\r\n", "0 1 -4 1\r\n", "0 4 0 -1 1 -1 0\r\n", "0 3\r\n", "-2 0\r\n", "1 -4 0 -2 0 4 0 -4 0 4 -3 0 1 -4 0 1\r\n", "0 -3 3 -2 0 3 0 -2 2\r\n", "1 0\r\n", "2\r\n", "0 -4\r\n", "0 4 0 -4 0 -3 3 -3 0 -2 0 -2 0 4 0 -1 1 0 3 0 -4 1 -4 0 4\r\n", "2 0 -1 1\r\n", "0 2 0 4 0 4 -4 0 -1 2\r\n", "0 3 -2 0 3 -2\r\n", "1 0 -3 3 0 -4\r\n", "0 -3 3 0 -1 0\r\n", "2 -2 0 1\r\n", "-4 1 -4 1 -4 0\r\n", "0 4 0 2 0 -4 1 2 -1 0 4 0 1 0 4 -4 4 0 -4 4 0\r\n", "-2 0 3 0 -2 0\r\n", "-2 2 -1 0 1 -4 0 3 -2\r\n", "1 -1 0 4 0 2 -2 3 0 1 -4 1 0 -3 4 0 3 0 4 0 4 0 -4 0\r\n", "-1 0 4 -4\r\n", "-1 0 -1 2 0 2 0\r\n", "-1 0 3 -2 0 2 -2 3 -2 2 -2 0 -3 4 0 1\r\n", "-2 2 -1 0 2 0 3 -1 3 -2 2 0 -2 2 -2 0 1 0 2 0\r\n", "1 -4 1 0 4 -4 0 2 0\r\n", "2 -2 0\r\n", "0 4 -4 -1 0 -1 1 -1 0 4 0 -2 3 -2 0\r\n", "-1 0 2 -1 0 4 -4 0 -4 0 4 0\r\n", "0 -3 0\r\n", "1 0 -1 2 -1 0 3 0 3 -2 3 -2 0 2\r\n", "2 0 2 0 -2 3 -2 2 -1 0 4 0 2\r\n", "-1 1 -4 1 0 1 0 -4 4 -4 0 3 -2 2 -1 0 3 0 -1 1\r\n", "2 0 -1 1 -1 0 3 -2 3 0 2 0 3 -2 0 -4 0 4 -4 0 4 0\r\n", "0 -1 0 3 0 2 -2\r\n", "1 -4 1 -1 0 2 0 3 -2 3 -2 3\r\n", "2 0\r\n", "-1 0 3 0 3\r\n", "1 -4 1 0 -4 4 -4 0\r\n", "-2 2 -1 0\r\n", "0 1 0 4 0 3 0 -2 0 3 0 4 0 2 -2 0\r\n", "0 3 -2 0 4 0 -2 2 -2 0 -2 0 4 0 -2 0 2\r\n", "2 0 1 -1 0\r\n", "1 0 -3 4 -3 0 -2 0 3 0\r\n", "0 3 -2 0 4 0 -3 3 0 3 -2 0\r\n", "2 0 3 0 1 0 3\r\n", "1 0 3 -3 0 4 -3 0\r\n", "-2 2 -2 0\r\n", "0 1 0 -3 4 0 3 -2 3 0 1 0 4 0 -1\r\n", "0 3\r\n", "-2 2 0 3 0 -2 0 2 0 -2 0 3 0 -4 0 -2\r\n", "0 3 0 -3 4\r\n", "0 3 -2 2 -2 3 -2 0\r\n", "-1 0 3 0 3\r\n", "2 0\r\n", "0 -3 0 1\r\n", "1 0 4 -4 1\r\n", "-2 2 0 4 0 -2 0 -2\r\n", "1 0 4 0 1 0 -3 3\r\n", "-2 2 0 3 -2\r\n", "1 0 -3 4 -3 0 3 0 3 0 -2 0 3 -2 0 1 -4 0 3 0 -2 0 3 -3 0\r\n", "-2 2 0 2 0 3\r\n", "0 3 -2 0 3 0 -4 1\r\n", "0 1 0 -4 4 0 -2 0 3 0 -4 0 4 0 -4 1 0 3 -2 3 0 -1 1 -1\r\n", "2 0 -3 4 -3 0 2 0\r\n", "0 3\r\n", "0 3\r\n", "-1 0 4\r\n", "0 3\r\n", "-2 3 0 1 -4 0 -2 2 -2 3 0 4\r\n", "2 -2 0 4 0 -4 1 -4 0 3 -2\r\n", "1 0 2\r\n", "0 3 0 2 -2 3 -3 0 1 0 -3 3 0 4 0 2 -2 2 -2 3 0\r\n", "2 0 -2 3 2\r\n", "0 1 0 4 -4 1 -1 2 -2 3 -3 0 -2\r\n", "0 -3 4 -3 0 2\r\n", "0 2 -2 3\r\n", "0 -4 0 -4 1 0 3 0 1 0 2 -2 0 -3 4 0 4 -3 0 3 -3 -2 0 -3 4 0 -4 0 3 0\r\n", "-2 2 -2 3 -3 0 -4 1\r\n", "0 -2 0 2 0 4 0\r\n", "0 -3 0 -4 0 -3 4 0 -2 3 -3\r\n", "2 0 -2 2 0 4 0 1 0 -2 3\r\n", "0 4 0 3 -2 3 0 -4 4 0 4 0 3 0 3\r\n", "2 0 -2 0 4 0 3 -2 2 -2 3 0 -2\r\n", "1 0 3 -3 0 3 0 3 -2 3 -2 3 0 3 0 -1 0 4 0 -4 1 0 3\r\n", "2 -2 0 -3 4 -3\r\n", "0 1 0 3 0 -2 2 -2\r\n", "1 0\r\n", "2 0 -2 3 -2 2 0\r\n", "1 0 -4 4 0 3 -2 3 -2 0 4 -3 0 -3 4 0 -4 1 -4 0 2 -2 0 3 -3 0 1 0 3 0 -2 3 0 4 0 -4 1 0 3 0 -3 4 0 2\r\n", "0 -3 4 -3 0 1 0\r\n", "0 3 0 4 0 -4 1 0 -2 0\r\n", "2 -2 0 -2 0 -4\r\n", "-1 0\r\n", "2 0 4\r\n", "1 0 3 0\r\n", "2 0 -4 4 0 1 0 3 -2 0 4 0 -4 0 3 0 -2 3\r\n", "0 2 -2 0 -4 0 -4 4 -3 0 -4 1 0 4 0 -3 3 0\r\n", "1 0 4 -3 0 2 -2 0 4 0 -3 4 -3 0 -4 0 -3 0 -4 1 0 -2 3 -2 0 1\r\n", "2 -2 3 0\r\n", "2 -1 0 4 0 1 0 3 -2\r\n", "0 3 0 -2 3 -2 0 -2 3 -2 2 -1 0 3 0\r\n", "1 0 1 0 4 -4 0 3 0 3 -2 0 4 0 3 -2\r\n", "0 3 -2 0 -1 1 0 2 -2 2 0 -3 4\r\n", "2 0 4\r\n", "0 -4 4 -4 0 1 -1 0 4\r\n", "-1 0 4 -4 0 -4 4 -4 0 2 0 -4 0 -3 3 -2 3 -2 0 -4\r\n", "2 0 -1 2 -1 0 1 -1 0 3 0 -2 0 3 0 -3 0 -3 0 -4 4 -4 1 -1 2 -1 1 0 3 0\r\n", "0 3\r\n", "1 0 -3 0 1 -4 0 2 0 -2 3 0 4 -4 0 -1 0 3 0 1\r\n", "0 -1 2 0 -3 4 0 -1 0 4 -4 4 -4 0 2 -1 1 0 -3 3 0\r\n", "0 3 -2 3 0 4 0 1 0 4 0 -4 4 -4 0 -4 4 -4 0 3\r\n", "2 0 3 0 1 0\r\n", "1 0 -4 1 -1 0 -2 -1 3 -2 2 -2 0 -3 0 1 -1\r\n", "2 0 3\r\n", "-4 1 -1 0 3 0 3 0 1\r\n", "0 4 0 -4 1 0 1 0 3 0 4 -4 0 -4 4 0\r\n", "2 0 -4 4 0 -1\r\n", "0 3 -2 2\r\n", "0 4 0 1 -4 4 -4 0 2 0 -3 4 0 4 -4 0 3 0 -1 1 -4 4 0 1\r\n", "0 1 -1 0 -4 0 4 0 1 0 4 0 2 0 -4 4 0 2 0 3 0 4 -4 0 3 0 4 0 -4 4\r\n", "1 0 -4 4 0 2 -1 0\r\n", "2 0 4 -4 1 -1 0 4 0 -2 2 0 4 -4 0 1 0 4 0 2\r\n", "0 4 0 3 -2 0 4\r\n", "0 3 0 -2 3 0 1 -4\r\n", "1 -4 1 0 -1 0 3 -2 2 0\r\n", "2 0 -1 0 3\r\n", "0 -1 0 2 0 -3 4 -4 0 3 0 1 -1 0 -4 4 -4 0 2 -1 1 0 3 0 4 -4 0 3 0 1 0 3 -2\r\n", "2 -1 0 3 0 4 -4 0 1 -4 1 -1 0 -4 4 0 -4 0 3 -2 0 4 -4 4 -4 0 2 -2 0 1 0 4 0 3 0 3 -2 3 -3 0 3 0 -3 0 1 -4\r\n", "1 -1 0 -2 3 -3 0 -4 0 -3 0 3 -2 0 3 -2 2\r\n", "0 4\r\n", "2 0 -2 3 0 2 -1 0 -3 0 -2 3\r\n", "1 0 3 0 3 0 -2 3 -2 0 -2 3 -2 0 3 0 1 -1 0 3 0 3 0 4 -4 0 1 -1 0 3 0 -3 0 -4 4 -4 0 3 0 -1 1 -4 1\r\n", "0 -1 2 0 3\r\n", "2 0 3 -2 0\r\n"]
  in  "CJ ALL":string[](array[string])=["0 3 0 1 0 -3 0 -3 3 0\r\n", "1 -4\r\n", "2 0 2 0 -1 0 -3\r\n", "0 4\r\n", "0 -1 2 -1 0 2 0 3 0 1 -4 1 0 -4 4 -4\r\n", "0 -1 0 -4 0 -2 0\r\n", "1 -1 1 0 -4\r\n", "-1 0 -4 0 1 0\r\n", "0 3\r\n", "-1 1 0 -4 1 0 -4 0 -1 2 0\r\n", "1 0 -1 0 2\r\n", "0 -1 -4 1 0 -3 3\r\n", "2 -1 0\r\n", "0 4 0 2 0 -3 0 1 -1 0 1 -4 4 -4 4 -4 0 3\r\n", "0 -4 4 -4 0 -1 2 0 3 -3 0 -3 3 0 -4 1 0 -3 0 3 -2\r\n", "0 3 0\r\n", "0 4 0 1 0 -4 4\r\n", "0 -1 0 4 0\r\n", "1 -1 0 4 0 2 -2 0 -4 1 -4 4 -3 0 -4 0 -3 3 0 -4 1 -1 2 -1 0 4\r\n", "0 3 0 4 -4 4 -4 1 -4 1 -4 4 -4 1 -4 0 -3 3\r\n", "", "0\r\n", "0 4 -4 0 -4 0 4 -4 0\r\n", "1 -4\r\n", "0 4\r\n", "0 1 -4 1 -4 0 -4 4 -4 0\r\n", "-2 2 0 -3 3 -3 0 3 0\r\n", "1 0 4 0\r\n", "0 3 0 1 0\r\n", "0 4 -4 0 -4 1 -4 0\r\n", "0\r\n", "0 -4 4 -4 0 -3 3 -2 0 2\r\n", "0 3 0 1 0 -4 4 0 -3 3 0 -4 0\r\n", "0 1 0 3 -2 3\r\n", "0 2 -2 3 -3 0 -3 3 -2 2 0 -4 4 -4 1 0 4 0 2 -2 0 4 0 4 0 2 -2 2\r\n", "0 -3 3 0 -2\r\n", "1 0 -2 0 4 0 1 0 -2 2 -2\r\n", "-2 0 3 0\r\n", "-4 0 -2 0 3 -3 0 -2 2 -2 0 -4 0 3 -2 0\r\n", "0 -3 4 0 1 0 -2\r\n", "-2\r\n", "-4 0\r\n", "-2 0 -3 4 -3 4 -4\r\n", "0 1 -4 0 -2 2 -2 0 -4 0 -3 3 -2 3 0 1 0\r\n", "0 3\r\n", "0 2 0 3 0 1 0 -2 2 -2 3 0\r\n", "-1 0 -1 1 0 4 -4 4 -4\r\n", "0 -3 4 -3 -2 2 -2 3 -2 2 -2 0\r\n", "2 0 -3 3\r\n", "0 3 0 -1 0\r\n", "0 3\r\n", "0 3 0 3\r\n", "-4 0 -4 1 -4\r\n", "2 -2 0 3 -3 0 1 0 -1 0 4 -3 0 2 -2 0\r\n", "0 1 0 4 -4 4 0\r\n", "0 1 0 -3 3 -3 0\r\n", "0 -3 4 0 -4 1 0 -2\r\n", "0 3 0 -2\r\n", "2 0 -3 3 -2 2 0 -2 0 -3 4 -3\r\n", "0 1 0 3 0\r\n", "0 3 0 -2\r\n", "-4 0 3 0 2 -1 0 3 0\r\n", "2 0 4 0 -2 2\r\n", "0 -3 4 -3 0 -2 2 -2 0 4\r\n", "0 3 -2 0 -3 4 0 3 0 1 -1 0 -1 0\r\n", "0 -3 4 -3 0\r\n", "2 0 3 -3 0 -4 0 -2\r\n", "-1 0 3 -3 0 1 0 4\r\n", "0 1 0\r\n", "0 -1 0 -1 1 -1 0\r\n", "0 -3 3 -3 0 1 -4 0 -1 0\r\n", "2 0 3 -2 0 -2 3 -2 0\r\n", "0 1 -1 1 -1 1 0\r\n", "1 0\r\n", "2 -2 0 3 0 4 0 -1 0 -1\r\n", "0 4 -4 1\r\n", "0 4 -4 0 4 0 -4 1 -1 0 -3 3 0 4 -4 0 -1 0 4\r\n", "-4 0 -3 0 -4 0 2 0 4 0 -2 0 -1 1 0 4 -4\r\n", "0 -1 1 0\r\n", "0 4 0 1 -1 0\r\n", "0 2 -1 0 -4 4 -4 0 -1 1\r\n", "2 0 2 0 2 0 -3 0 4 -4 1 0\r\n", "1 0 4 0 2 0 -2 3 -2 0 4 -4 0\r\n", "0 4 0 2 0 4\r\n", "-1 1 -1 2\r\n", "0 4 -4 0 -1 2 0 -4 1 -4 4 -4 0 -4 4 -3 0 4 -4 1 0 3\r\n", "0 -1\r\n", "2 0 2 0 2\r\n", "0 3 -2 0 -1 1 -1 0 -3 0\r\n", "2 0\r\n", "0 3\r\n", "0 4 -4 1 0 3 -2 2 -2 2 0 4 0 4 0\r\n", "-4 0 -2 0 2 0 4 -4 1 -4 1 0 1\r\n", "0\r\n", "0\r\n", "0 4\r\n", "-2 2 0 -1 0 4 -4 1 0 1 -1 0 1 0 4 0 -4 4 0 2 0\r\n", "0 -1\r\n", "1 0 4 0 -2 0 -2 0 1\r\n", "2 0 -4 0 4 -3 0 1\r\n", "0 -1 1 0 -4 0\r\n", "-4 1 0 -4 0 -1 1\r\n", "0 4 0 2\r\n", "0 3 2 3\r\n", "2 0 -4 1 -4 4 -3 0 2 -1 1 -1 0 4 0 -3 0 2 0 3 -2 2 0 3\r\n", "0 1\r\n", "2 0 3 -3 0 3 -3 0 4 0 4 0 -2 0 3\r\n", "0 -1\r\n", "0 4 0 3 0\r\n", "-4 0\r\n", "0 3 0 2 0\r\n", "0 1\r\n", "-2 0 -3 3 -2 0 3 -3 0 -4 4 0 1 0 -2 3 0 -3 4 0 1\r\n", "0 -1 2 0\r\n", "-4 0 4 -4 0 -2\r\n", "0 -1 0 4 -3 0 2 -2 3\r\n", "0 3 0 1 0 3 -3 0 1 0 1\r\n", "2 0 3 0 2 0 -3 4 0 -3 4 0 2 0 3 0 2\r\n", "0 3 0\r\n", "-4 0 2\r\n", "0 1 0 1 -4 4 -3 0 3 -3 4 0 2 -2\r\n", "0 4 0 2 -2 0\r\n", "0 4 0\r\n", "0 1 -4 4 -4 0 -3 3 0 -2 3\r\n", "0 1 -4 0 -4\r\n", "0 2 0 4\r\n", "0 -1 0 4\r\n", "-4 0 -2 3\r\n", "0 3 0 1 -4 0 -4\r\n", "0 1 -1 2\r\n", "0 3 -3 0\r\n", "0 4 0 -1 2\r\n", "-4 0 -4 4 0 4 0 -4 4\r\n", "0 3 -2 0\r\n", "0 3 -2 3 -2 2\r\n", "0 1 0 4\r\n", "0 2 -1 0 -1 0 -4 4 -4 1 0 1 -4 1 0 -1 1 -4\r\n", "1 0 -1 0 4 -4 1 -4 1 0 4 -4 -1 0 -1\r\n", "0 -3 3 0 2 -1 0\r\n", "0 -1 2 0 -3 -4 1 0 1\r\n", "2 -1 0 -2 2 0 3 -2 0 -4 4 -4 0 4\r\n", "0 3 0 -3 0 1 0 -4 4\r\n", "0 2 -1 0 2 0 4\r\n", "0 4 -4 0 2\r\n", "0 1 0 3 0 -1 0 -4 0 1 -4 0 -4 0 3 0 -4\r\n", "-4 1 -4 1\r\n", "0 -1 0 4 -4 1 -4 1 0 3 0 3 0 -4 0 -4 0 4 -4 1\r\n", "0 1 0 1 -4 1 0\r\n", "0 2 0 -4 0 -1 2 -1 0 4 -4\r\n", "1 -4 1 0 4\r\n", "0 3 -2\r\n", "2 0 -1 0\r\n", "0 2 0 -2 0\r\n", "0 4 -4 1 -4 1 0 4 -4 1\r\n", "0 3 0 -2 2 -2 2 0 4\r\n", "-3 0 -1 0 -3\r\n", "0 1 -1 0 1 0 -4 1 0 -4 4 0 2 0 4 0 -3 3 0 4 -4 1 -4 1 0 4\r\n", "-3 0 4 0\r\n", "-4 1 0 -1 0 -1 0 -2 0\r\n", "0 3 0 -1 2 -1 0 4 -4 0 -3 0 -1 1 0 2\r\n", "0 1 0 1 -4 1 0\r\n", "0 2 -1\r\n", "1 -4 1 0 4\r\n", "0 4 0\r\n", "0 2 -1 0\r\n", "0 3 -2 0 4 0 4 -4 0 2 0\r\n", "-1 0 -3 3 0 1 0 4\r\n", "0 1 0 1 0 4 0 -2 2 0 4 0 -2 0 1 0 3 0 3\r\n", "-4 1 0\r\n", "2 0 -1 0 4 -3 0 3 0 -2\r\n", "-4 0 4 0 -4 1 0 -4 0 -4 4 0 3 0\r\n", "0 3 -3 0 2 -2 0 -4 4 -4 0 -3 3 0\r\n", "0 -2 2 -2 0 3\r\n", "0 -4\r\n", "0 2 -2 0 2 0 -2\r\n", "-4 1 0 4 0 -2 2 -2 0 -2 3 -2 0 1 0 1 0 3\r\n", "0 2 0\r\n", "0 -3 3 -3 0 3 0 1 -4 0 3 0\r\n", "0 -3 4 0 1 -4\r\n", "0 3 0 -2 0 2 -1 0 2 -2 0\r\n", "0 4 -3 0 2 0 4 -3 0 -2 2 -2 0 -2 0 4\r\n", "-4 0 1\r\n", "0 -3 0 -3 0 4 0\r\n", "-1 0 1 0\r\n", "0\r\n", "0 3 0 3 -3 0 3 -3\r\n", "0 -3\r\n", "0 -4 4 -4 0 3 0 4 -4\r\n", "0 4\r\n", "1 0 1 -4 1 -4 1 0 2 -2 2 0 -4 0 -2 3 0 -1 1 0 4 -4 1\r\n", "0 -3 3 0\r\n", "2 -1 0 4 -1 4 -4 0 -1 1 0 -3 0 -4 1\r\n", "-4 0 -4 0\r\n", "-1 0 -1 0 4 0\r\n", "0 -3 3 0 2 -2 2 0 -3 0 1 0 1 -4 4 -4 1 0 3 -2 0 1 -1 0\r\n", "0 1 0 2\r\n", "0 4 -4 1 -4 1 -4 1 -4 0 -3 3 0 2 0 -4\r\n", "-4 1 0 2 -2 0 -2 3 0 1 0\r\n", "0 -3 3 0 -1 1 0 -1 0 4 0 -3 4 -4 1 -4 0\r\n", "0 1 0 3 -3 0 -2 3 -3 0 4 -4 0\r\n", "0 4 -4 0 -1 0 3 -3 0 -4 0 1 0 -4 4 -4 1\r\n", "0 1 0 4 -3 0 2 -1 0 4 0 -4 4 -4 0 -4 4 -4 0 4 0 1 0 3 0 -2 3 -2 0 3 -3 0 1 0 4 0 -2\r\n", "0 1 -1 0\r\n", "0 -1 0 3 0 -4 4\r\n", "0 -3 0 -2 2 0 -1 1\r\n", "0 4 -4 0\r\n", "0 -3 3 0 3 -3 0 -4 4 -4 0 4 -4 1 0 2 0 -2 3 -2 0 3 0 4 -4 0 2 -2 0 1 -4 4 -4 0 3 0 2 -1 0 1 -4 1 0 3 -2 0 3 0 1\r\n", "1 0 1 0 2\r\n", "0 3 -3 0 2 -2 0 3 -2 0 4 -4 1\r\n", "0 4 -4 0 -1 0 -3 3 0\r\n", "0\r\n", "0 4 0 -4\r\n", "0 -1 2 -1 0 3\r\n", "0 3 0 -2 2 0 -3 3 -3 0 4 0 3 -2 2 0 -4 4 -4 4 -4\r\n", "-4 1 -4 1 -4 4 -3 0 3 0 -2 0 4 0 3 0 1 -4 0 -4 4 -4\r\n", "0 3 0 -4 4 -3 0 -2 0 4 0 3 0 2 0 2 0 4 0 -4 4 -4 0\r\n", "0 1 0 -4 4 -4 0 -1\r\n", "0 2 -2 0 3 -3 0 -4 4\r\n", "-4 0 4 0 4 0 -4 0 -2 2 0 4\r\n", "0 -3 3 0 3 0 3 -3 0 4 -4 0 -4 0 3 -3 0\r\n", "2 0 4 0 3 -3 0 1 0\r\n", "0 4 -3 0\r\n", "-4 0 3 -2 0 1 0 -2\r\n", "0 -1 1 0 3 0 4 0 -2\r\n", "0 4 0 -3 3 0 2 0 4 -4 1 -4 0 -3 3 0 3 0 2 0\r\n", "0 4\r\n", "0 3 -3 0 -3 3 0 3 0 -3 4 0 4 -4 0 2\r\n", "-4 1 0 4 -3 0 3 0 4 -3 0 2 0 4\r\n", "-2 0 1 -4 0 4 -3 0 2 -2 0 3 0 3 0 -2 2 0 4\r\n", "0 1 0 -2 0 4 -4 0\r\n", "0 4 -3 0 -1 1 0 1 0\r\n", "0 3 -3 0\r\n", "0 2 -1 0 4 -4 0 3 0 2 -2\r\n", "-4 1 0 3 0 -3 4 0 2 -2 3 -2 2 -2 0 1\r\n", "0 3 0 -2 0 -4 0\r\n", "-2 2 0\r\n", "-4 1 0 -2 0 3 0 1 0 3 0 3 0 4 0 -2 0 -2 2 -2\r\n", "-2 0 -3 4 -3 0 2 -2 3 -2 0 -2 2 -2 0 4 -3 0 3 -3 0 1 0 3 -3 0 4 -3 0\r\n", "0 3 0 -4 0 2\r\n", "0 -4 0 -2 0 -1 1 0 3 -3 0 1 0 3 0 -2 0 3 0 4 0\r\n", "-4 0 1 0\r\n", "2 0 4 0\r\n", "0 2 0\r\n", "0 2 0\r\n", "0 3 0 1 0 3 -3 0 4 0 -2 2 0 -4 0 -1 2 0 -3 4 0 -2 0 3 0 -2 0 -1 1 0\r\n", "0 2 0 4 0 2 0 3 0 -3 0 2 0 3 0 1 -4 0 -2 0 3 0 4 -3 0 2 -2 0 -2 0 4 0 -4 0 -4 1 0 2 0 4 -4 1 -1 0 2\r\n", "0 1 -4 0 2 -1 0 3 -3 0 -4 1\r\n", "0\r\n", "0 4 -3 0 -1 2 -1 0 4 0\r\n", "0 4 0 2 0 4 0 4 0 4 -4 0 -2 2 0 3 0 2 0 2 -2 0 -2 3 -2 0 1 0 1 0 2\r\n", "0\r\n", "0 2 0 4 0 -2 0 1\r\n"]
  in  "CJ top vs WF":string[](array[string])=["0 -4 4 -4 0 3 0 4 -4\r\n", "0 4\r\n", "1 0 1 -4 1 -4 1 0 2 -2 2 0 -4 0 -2 3 0 -1 1 0 4 -4 1\r\n", "0 -3 3 0\r\n", "2 -1 0 4 -1 4 -4 0 -1 1 0 -3 0 -4 1\r\n", "-4 0 -4 0\r\n", "-1 0 -1 0 4 0\r\n", "0 -3 3 0 2 -2 2 0 -3 0 1 0 1 -4 4 -4 1 0 3 -2 0 1 -1 0\r\n", "0 1 0 2\r\n", "0 4 -4 1 -4 1 -4 1 -4 0 -3 3 0 2 0 -4\r\n", "-4 1 0 2 -2 0 -2 3 0 1 0\r\n", "0 -3 3 0 -1 1 0 -1 0 4 0 -3 4 -4 1 -4 0\r\n", "0 1 0 3 -3 0 -2 3 -3 0 4 -4 0\r\n", "0 4 -4 0 -1 0 3 -3 0 -4 0 1 0 -4 4 -4 1\r\n", "0 1 0 4 -3 0 2 -1 0 4 0 -4 4 -4 0 -4 4 -4 0 4 0 1 0 3 0 -2 3 -2 0 3 -3 0 1 0 4 0 -2\r\n", "0 1 -1 0\r\n", "0 -1 0 3 0 -4 4\r\n", "0 -3 0 -2 2 0 -1 1\r\n", "0 4 -4 0\r\n", "0 -3 3 0 3 -3 0 -4 4 -4 0 4 -4 1 0 2 0 -2 3 -2 0 3 0 4 -4 0 2 -2 0 1 -4 4 -4 0 3 0 2 -1 0 1 -4 1 0 3 -2 0 3 0 1\r\n", "1 0 1 0 2\r\n", "0 3 -3 0 2 -2 0 3 -2 0 4 -4 1\r\n", "0 4 -4 0 -1 0 -3 3 0\r\n", "0\r\n", "0 4 0 -4\r\n", "0 -1 2 -1 0 3\r\n", "0 3 0 -2 2 0 -3 3 -3 0 4 0 3 -2 2 0 -4 4 -4 4 -4\r\n", "-4 1 -4 1 -4 4 -3 0 3 0 -2 0 4 0 3 0 1 -4 0 -4 4 -4\r\n", "0 3 0 -4 4 -3 0 -2 0 4 0 3 0 2 0 2 0 4 0 -4 4 -4 0\r\n", "0 1 0 -4 4 -4 0 -1\r\n"]
  in  "WF bottom vs CJ":string[](array[string])=["2 -2 0 4 0 -4 1 -4 0 3 -2\r\n", "1 0 2\r\n", "0 3 0 2 -2 3 -3 0 1 0 -3 3 0 4 0 2 -2 2 -2 3 0\r\n", "2 0 -2 3 2\r\n", "0 1 0 4 -4 1 -1 2 -2 3 -3 0 -2\r\n", "0 -3 4 -3 0 2\r\n", "0 2 -2 3\r\n", "0 -4 0 -4 1 0 3 0 1 0 2 -2 0 -3 4 0 4 -3 0 3 -3 -2 0 -3 4 0 -4 0 3 0\r\n", "-2 2 -2 3 -3 0 -4 1\r\n", "0 -2 0 2 0 4 0\r\n", "0 -3 0 -4 0 -3 4 0 -2 3 -3\r\n", "2 0 -2 2 0 4 0 1 0 -2 3\r\n", "0 4 0 3 -2 3 0 -4 4 0 4 0 3 0 3\r\n", "2 0 -2 0 4 0 3 -2 2 -2 3 0 -2\r\n", "1 0 3 -3 0 3 0 3 -2 3 -2 3 0 3 0 -1 0 4 0 -4 1 0 3\r\n", "2 -2 0 -3 4 -3\r\n", "0 1 0 3 0 -2 2 -2\r\n", "1 0\r\n", "2 0 -2 3 -2 2 0\r\n", "1 0 -4 4 0 3 -2 3 -2 0 4 -3 0 -3 4 0 -4 1 -4 0 2 -2 0 3 -3 0 1 0 3 0 -2 3 0 4 0 -4 1 0 3 0 -3 4 0 2\r\n", "0 -3 4 -3 0 1 0\r\n", "0 3 0 4 0 -4 1 0 -2 0\r\n", "2 -2 0 -2 0 -4\r\n", "-1 0\r\n", "2 0 4\r\n", "1 0 3 0\r\n", "2 0 -4 4 0 1 0 3 -2 0 4 0 -4 0 3 0 -2 3\r\n", "0 2 -2 0 -4 0 -4 4 -3 0 -4 1 0 4 0 -3 3 0\r\n", "1 0 4 -3 0 2 -2 0 4 0 -3 4 -3 0 -4 0 -3 0 -4 1 0 -2 3 -2 0 1\r\n", "2 -2 3 0\r\n"]
  in  "DU top vs CL":string[](array[string])=["0 -1 0\r\n", "0 3 0 4 0\r\n", "0 2 0 -1 0 3 0 -1 0 -1 0 1 0 1\r\n", "0 -1 0 -2 -1 1 0 -3 0 3 0 2 -1 0 3 0 1 -4 4 0 4 -4 1 -4 4\r\n", "0 3 0 3 0 4 0 2 -2 0 4 -4 0 2 0 1 -4 4 -4 0 3 0\r\n", "0 -1 0 4\r\n", "1 0\r\n", "2 0 4 -4 0 1\r\n", "-4 1 -1 0 2 0 1 -4 0 -3 0 2 -2 0 4 0\r\n", "0 -1 0 3 0\r\n", "0 3 0 1 0 1\r\n", "0 -1 0 4 -4\r\n", "1 -1 0\r\n", "0 3 0 4\r\n", "2 0 -2 3 -2 0 4 0 -4 1 -4\r\n", "0 -1 0 3 -2\r\n", "0 -3 3 0\r\n"]
  in  "CL bottom vs DU":string[](array[string])=["0 1 0\r\n", "2 0\r\n", "0 1 -4 0 -4 0 -3 4 -4 0 2 0 2\r\n", "0 3 -2 2 0 -4 0 -3 0 1 -4 4 0 2 0 -3 3 -3 0 -2 2 0\r\n", "0 2 0 3 -3 0 3 -3 0 1 0 4 -3 0 2 0 -2 0 4 -4 1 -1\r\n", "-4 1 0\r\n", "0 2 0\r\n", "0 1 0 -4 0 -4 0 -1 0\r\n", "0 4 -4 0 -4 4 -3 0 2 0 -1 1 -1 0 3\r\n", "0 2 0 -4\r\n", "0 3 -2 0 -2 0 -2 3 -2 2 -2 3\r\n", "0\r\n", "0 -3 4 0\r\n", "0 2 0\r\n", "0 -3 4 -3 0 -2 2\r\n", "0\r\n", "0 2 0 1 0 -3 4\r\n"]
  in  "CL top vs DU":string[](array[string])=["2 0 -4 1 0 3 0 -4 1 -1 0 4 -4 1 0 2 -2\r\n", "1\r\n", "2 0 -1 0 -1\r\n", "1 0 4 -4 0 2 0 -1 0 -1 0 4 -4 0 2 0 3 -2 3 0 -1 1 0 4\r\n", "0 1 0 -2 0 -1 1 -4 4 0 -4 0\r\n", "0 -1 0 -1 0\r\n", "2 0 -1 1 0 4 -4 1 0 1 0 -3 0 -2 0 -4 0 4 0 1 0\r\n", "0 4 -4 1 -4 1 -4 0 -1 0 -1 0 -1 1 0 -4 4 0 -1 0\r\n", "0 3 -2 0 3 0 2 0 2 0 -4 1 0 -3 0 1 0 4 -4 0 3 -3 0 1 0 -1 0 -1 -4 4 0 2\r\n", "1 -4 1 -1 0 -4 1\r\n", "2 -1 0 -4 1 0\r\n", "1\r\n", "2 0 1 0 -4 1 -4 4\r\n", "0 2 0 -2 2 -1 0 4 -4 0 -4 4\r\n", "1 0\r\n", "2 0 -4 4 0 2 -1 0 -4 4 0 1 -1 0 4 0 2\r\n"]
  in  "DU bottom vs CL":string[](array[string])=["0 3 -2 0 -2 0 -2 0 -2 2 -2 0 3 -3 0 2 0 -3 4 -3 0\r\n", "0\r\n", "0 3 -3 0\r\n", "0 2 -2 0 3 -3 0 1 -4 -1 1 0 -4 0 3 0\r\n", "-4 1 0 2 -1 0 3 -3 0 -4 0 2 0 3 0 -4 1\r\n", "0 2 0\r\n", "0 3 -2 0 3 -3 0 3 0 2 0 3 0 3 0 -2 2 -2 0 -2 3\r\n", "-4 1 0 -2 3 0 -1 0 3 0\r\n", "0 1 -4 0 -4 0 3 0 2 -2 0 4 -4 1 0 3 -3 0 -2 3 0 -4 0 2 0 -4 0\r\n", "0 -4 4 -3 0 3\r\n", "0 3 -2 3\r\n", "0\r\n", "0 -3 3 -3 0 2 0 3 0 -2 2\r\n", "-4 1 0 3 0 -3 -2 3 0 1 -4 0 3 -3 0 1 0 -2 0 2 0\r\n", "-1 0 -2 3 -2 0\r\n", "0 3 0 3 -3 0 -4 0 -3 3 -3 0 -4 0 4 -3 0 1 -4\r\n"]
  in  "DU top vs CL":string[](array[string])=["0 -1 0 4 0 -1 0 1 -4 4 -4 1 0 -4 1 -4 0 1 0 4 -4 0\r\n", "0 -2 0 2 0\r\n", "1 -1 0\r\n", "0\r\n", "-1 0 3 0 4\r\n", "0 2 0 4\r\n", "0 -1 0 -4 0 1 -4 1 0 -4 1 0 3 0\r\n", "1 -1 0 -4 0 -3 4 0 -1 0 3 -2 2 0 -3 0\r\n", "0 -1 0 2 0 3 0 2 0 4 0\r\n", "0 3 0 1 -1 0 -1 2 -1 0 1 -4 1 0 2 0 3 0 -4 0 2 0 1 0 2 0 -2 0 1\r\n", "2 0 -2 3 0 -1 0 -1 0 -1 0 3 0 2 0 4\r\n", "0 3 -2 0 1 0 -1 0\r\n", "0 -4 4 0 2 -1 0 1 0 1 0 3 0 4 0 -4 4 -4 0 -4 0 -1 2 -1 0 1 -4 1 0 -2 0\r\n", "0 3 0 3 -2 0 -4 0 -4 0 3 0 1 0 -2 3 0 -4 4 -4 0 2 0 3 0 -4 4 -4 0 2 0 4 -4 0\r\n", "1 -4 1 -4 4 -4 1 -4 1 -4 0 -3 3 0\r\n", "2 -1 0 4 -4\r\n", "1 0 3 0 2 0 -4 1 0 -2 0 -2 3 0 1 -4 1 0 3 -2 2 -1 0 -3 4\r\n", "0 3 -2 0 -1 0 3 0 -2 0 -4 4 0\r\n", "-1 0\r\n", "-1 0 -2 0\r\n", "1 -1 0 3 0 1 0 1\r\n", "2 0 2 0 -2 3 -2 0 -1 0 3 0 1 0 3 -2 -1 0 4 0 2 -1 1\r\n", "1 0 -2\r\n", "2 -1 0 -1 0 4 0\r\n", "0 3 0 1 -4 0 -1 0 3 -2 0 1 -4 1 0 1 0 3 0 -4 1 0 3 0\r\n", "-1 0 3 0 3 0\r\n", "1 -1 0 3 -2 0 -1 0 -1 0 3 -2 2 0 3 0 2 -2 0 3 0 -2 0\r\n", "0 3 0 4 -4 1 -4 1 0\r\n", "0 -1 0\r\n", "0 3 0 4 -4 0 3 0\r\n", "-1 0 3 -2 0 1 0\r\n", "0\r\n", "-1 0 4 0 2 0 -2 3\r\n", "2 -1 0 4 -4 0 -1 0\r\n", "-4 1 0 -1 0 -1 0 -4 4 -4 0 -1 0 -4\r\n", "2 -1 0 3 -2 0 1 -4 1 0 -2 0 1 -1 0 -2\r\n", "0 3 -2 2 0 3 -3 0 1 -4 1 0 -2 0 4 0 -4 1 -4 0 3 0 1 0 4 -4 0 -4 4 -4\r\n"]
  in  "CL bottom vs DU":string[](array[string])=["0 1 0 -3 4 -3 0 2 -2 0 -2 0 -3 4 -3 0 -2 2 -2 0 -3 4 0 2 0\r\n", "-4 0 -4 4\r\n", "0 4\r\n", "0 2 0\r\n", "-4 0\r\n", "0 -3 0\r\n", "-2 2 0 -3 3 0 3 -3 0 -2 2 -2 3 -3 3 -2 0 -3 4 0 4\r\n", "0 -3 3 0 2 0 -4 1 0\r\n", "-4 1 -4 4 0 1 -1 0 3\r\n", "0 -3 4 0 -3 3 -3 0 -2 0 -4 0 -2 0 -3 3 0 1 0 -4 4 0 -3 3 0 3\r\n", "0 4 0 -4 0 -1 0 1 -4 4 -4 0\r\n", "0 1 0 -3 4 0 2\r\n", "0 2 0 3 -3 -4 1 -4 4 -3 4 0 -4 0 -3 4 -3 0 -2 2 0 -4 0 3 -2 3 -2 0 -3 3 0\r\n", "-4 1 0 -4 0 3 -2 0 -3 4 0 2 0 3 -3 0 1 -4 0 2 -2 0 -2 0 -3 3 0 3\r\n", "0 -2 2 -2 0 -2 2 0 3\r\n", "0 -3 3 0 3\r\n", "0 2 0 4 0 2 -2 0 -3 4 0 1 -4 0 -2 2 0 -4 1 0\r\n", "0 -3 3 -3 0 1 0 3\r\n", "0\r\n", "0\r\n", "0 4 0 -2 0 -3 4 -3 0\r\n", "0 1 -4 0 -4 0 2 -2 3 0 2 0 1\r\n", "0 3 0\r\n", "0 -3 3 -3 0 3\r\n", "0 3 0 4 -4 0 -3 3 -3 0 2 0 2 0 4\r\n", "0 4\r\n", "0 2 0 -4 0 1 0 1 -4 0 4 0\r\n", "0 2 -2 0 3\r\n", "-4\r\n", "2 0 1 -4 0 4\r\n", "0 4 0\r\n", "2\r\n", "0 1 -4 0 4 -3 0 -4\r\n", "0 2 0 3\r\n", "0 2 0 -3 3\r\n", "0 2 0 -2 2 -2 0 -3 4 -4 1 0 -3 4 0\r\n", "0 -4 0 -4 1 0 2 0 2 0 3 -3 0 -4 1 0 3 -2 2 0 -3 4 -3 0 3 0 3\r\n"]
  in  "CL top vs DU":string[](array[string])=["0 4 -4 1 -4 0 -4 1 -4 4 -4 0 1 -1\r\n", "0 -1 1 0 -4 0 -1 0 3 -2\r\n", "1 -4 1 0 1 -4 4 -4 1 0 1 -4 1 0 4 0 4 -4 0 4 -4 1 0 4\r\n", "2 0\r\n", "1 0 1 0 -3 0 -3 3 -2 2 -1 0 -1 0 -1 0 -4 1 0 2 -2 2 0 4 -3 0 4 -4 1 0 4 0 -1 2 0 -3 0 3 0 1\r\n", "2 0 2 0 -4 4 -4 0 -4 4 -3 0 2\r\n", "0 3 0 2 -1\r\n", "0 4 0 -2 0 3\r\n", "0 4 -4 1 0 -4 0 4 -4 0 2 0 -1 1 -1 0 -1\r\n", "1 0 4 -4 1 0 4 -4 0\r\n", "2 -1 0 -1 0 4\r\n", "1 -4 1 0 4 0 2 0 2 0 -3 0\r\n", "2 -1 0 -3 0\r\n", "0 -1 1 0 1 -4 4 -4 0 -1 0 -3 3 0 1 0\r\n", "0 2 0 3 0\r\n", "1 0 1 -4 1 0\r\n", "2 0 3 0 3\r\n", "0 3 0\r\n", "0 2 0 3 0 3 0 3 -2 0 1 -4 1 -4 4 -4 1 -4 4 -4 4 -4 1 -4 0 -2 0 1 0 -4 4 -4 0\r\n", "0 4 0 -2 0 1 -4 4 -4 1\r\n", "0 4 -4 1 -4 1 0 1 -4 1 -4 1 -4 0 2 0 3 0 2 0 -3 3 0 3 -2 0 -1 1\r\n", "1 0 1 -4 1 0 -1 0 -4 0 -1 0 4 0 4\r\n", "0 1 0 1 0 1 -4 1 -4 4 0 -1 0 3 0 -1 0 4 0 2 0 2 0 4 -4 4\r\n", "0 2 0 1 0 -4 1 0 4\r\n", "2 0 -1 0 2 0 4 0 -2 0 3 0 2 0 2 -2 2\r\n", "0\r\n", "0 2 0 -2 0 -1 1 -1 0 -4 1 -4 1 -4 1 0 -4 4 0 -4 0\r\n", "1 0 -1 0 1 -4 1\r\n", "2 -1\r\n", "0 1 0 3 0 1 0 4 0 4 -4 1\r\n", "0 4 0 2 0 1 0 1 0\r\n", "-4 1 0 -4 0 -2 0 2 -1 0 4 -4 1 0 4 -4 0 2 0\r\n", "0 -3 3 0 1 0 1 0 -4 4 -4 0 1 0 4 -4\r\n", "2 0 1 0 1 0 2 0 3 -2 3\r\n", "0 4 0 2 0 -2 2 0 -4 4 -4 0 3 0 4 0 2 -1 0 4 -4 0 -4 4 0 2 0 -2 3 -2 2 -1 0 -4 4 -4 0 2 0 -3 0 -3 3 0 4 -4 0 2 -1 1 -4 4 0 2\r\n", "1 0 -4 1 -4 0 -4 4 0 -1 0 -4 1 0 1 -4 1 -4 1 -1 0 4 -4 0 3 0 -1\r\n", "0 -3 3\r\n"]
  in  "DU bottom vs CL":string[](array[string])=["-4 0 -2 0 3 -3 0 -3 3 0 -4 0 2 0 -4 0 2 -2 0 -3\r\n", "0 3 0 -3 4 0 2 0 3 -3 0 -4\r\n", "0 3 -2 0 4 0 -2 0 3 -3 0 3 0 3 -3 0 -2 0 4 -3 0\r\n", "0 4 0\r\n", "0 2 0 -4 0 -4 0 3 -2 0 -3 3 0 2 -2 3 -3 0 -4 1 0 -4 0 -2 0 4 0 -2 0 -2 0 1 0 4 0 -2 2 -2 0 3\r\n", "0 4 0 -2 2 0 3 0 -4 1 -4 0\r\n", "-4 0 -4 0 -4 0 -3\r\n", "0 4 -4 1 -4\r\n", "-4 0 -2 3 -2 3 0 -4 4 -4 4 -4 0 4\r\n", "0 3 0 -2 0 1 0 4\r\n", "0 3 0 2 0\r\n", "0 3 0 -4 0 3 -3 0 -4 1 0 4\r\n", "0 4 -4 4 -4 0 -1 0\r\n", "-2 0 3 0 -4 0 -2 2 0 3 -3 0 -2 2 -2 -3 3 -3\r\n", "-4 0 -3 0 3 -2 0 3 -2 2 -1 0\r\n", "0 3 -3 0 1 -4 0\r\n", "0 2 0\r\n", "0\r\n", "-4 0 4 0 -4 0 -4 4 0 2 0 4 -3 0 2 -2 0 -2 3 0 -2 2 -2 0 -2 0 -2 3 -3 0 4 0 4 -4 1 0 -3 3 0 -4\r\n", "0 -2 3 0 -4 1 -4 0 -2 2 -2 0 -2 3 -3\r\n", "-4 0 -2 3 0 2 -2 3 0 3 -3 0 -3 3 -3 0 3 -3 4 0 2 0 4 0 -4 0\r\n", "0 3 0 3 0 -1 2 0 3 -3\r\n", "0 3 -3 0 2 0 3 -3 0 -3 3 -2 0 1 0 1 0\r\n", "-4 0 -3 3 -2 2 -2 0 3 -3 0 -2 2 0\r\n", "0 3 -3 0 -4 1 0 4 0 -3 3 -3 0 -4 1 -4 0\r\n", "0 2 0\r\n", "-4 0 4 -4 4 -4 0 4 0 2 0 3 0 3 -2 2 0\r\n", "0 3 -2 0 3 0 -2 2 0\r\n", "0\r\n", "0 3 -3 0 -4 0 -4 0 -2 0\r\n", "-4 0 -4 0 -3 3 0 3 -3 0 -4 1 0\r\n", "0 3 0 -3 4 -4 1 -4 0 -3 3 -3 0 -2 2 0 1 0 -2 0 -4 1\r\n", "0 2 -2 3 -3 0 4 -4 4 0 2 0 3 -3 0 -2 0 1 0\r\n", "0 3 -2 0 3 -3 0 1 -4 1 0\r\n", "-4 0 -4 0 3 0 3 0 3 0 2 0 -2 0 -2 0 -3 3 -3 0 1 0 3 -3 0 -2 0 4 0 -4 0 -2 3 0 -4 1 -4 1 0 4 0 -2 2 0 -4 0 3 0 -4\r\n", "0 3 0 3 0 -2 0 3 -3 0 3 0 2 0 -3 4 -4 1 0 3 -3 0 1 0\r\n", "0 2 0\r\n"]
  in  "WZ top vs CL":string[](array[string])=["-2 2 0 2 -1 0 4 0\r\n", "1 -4 1 0 -4 0 3 0 -1 0 -4 0 2 -2 0 4 0 2 0 4 -4 0 2 -2 0 1 0 -4 1 0 4 -4 0 1 -4 1 0 4 -4 0 2 0 4\r\n", "-2 2 0 -1 0\r\n", "0 -1 0 -1\r\n", "4 1 -1 0 4 -4 0 -1 0\r\n", "0 -2 2 0 -2 2 -2 0 4 -4 0 -1 0 -1\r\n", "0 -4 4 -4 -1 0 -1 0 1 -4 4\r\n", "-4 1 0 -1 0 -1 0 4 -4\r\n", "2 -1 0 1 0 4 -4 0 2\r\n", "0 1 0 4 -1 4 -4 1\r\n", "0 -1 0 4 0 -1 0 -1 0 2 -2\r\n", "-4 1 -4 1 0 1 0 -1 0 4 -4 0 2 0 3 -2 0 1 0 1 0 -1 2 -1 0\r\n", "-2 2 0 -1 2 -1 0 -3 3 0 -1 0 4 0 1 -4 0 -4 0 4 0 2 0\r\n", "1 0\r\n", "-2 2 -2 2 0 -3 0 1 -4 1 0 1 -4 1 -4 0 -3 3 0 4 0 1 -4 4 0\r\n", "1 -4 1 0 -4 1 0 -4 1\r\n", "0 -1 2 -2 2 0\r\n", "2 0\r\n", "-4 1 -4 1 0 -3 0 -1 0 1 -4 1 0 -1 1 -1 0 1 0 1 0 4 -1 4\r\n", "0 -4 0 1 -4 0 1 0 1 0 -3 3 0 2 -2 2\r\n", "-2 2 0 -1 0 -3 4 0\r\n", "0 1 -1 0 4 -4 1\r\n", "1 -4 1 0 4 -4 1\r\n", "0 4 -4 0 -1 0 -2 0 -1 0 -1 0 -3 3 0 -1 0 -1 0 -1 0 2 0 4 -4 1\r\n", "-2 2 0 2 -1 0 4 -4 0 -4 4 -4 -1 -4 1 0 -4 4 -4 0 2 -2 3 0 1 0\r\n", "1 -4 1 -4 0 -3 0 3\r\n", "0 -1 0 1\r\n", "0 -1 0 -1 0 -3 4 0 -4 0 -1 2 -1 0\r\n", "0 2 0\r\n", "1 -4 1 0\r\n", "2 0 4\r\n", "0 -1 0 -3 -1 -3 0 1 -4 0 -4 0 -3 0 1 -4 0 3 -2 -1 0 -4 1 0 -4 0 4 -4 0 2\r\n", "0 -1 0 1 0 -1 2 -1 0 -2 0 4\r\n", "0 -1 0 1\r\n", "0 1 -4 1 0 -1 0 -3 -1 -3\r\n", "0 -1 1\r\n", "0 -1 0 3 0 1 -4 1 0 4 0 -4 1 0\r\n"]
  in  "CL bottom vs WZ":string[](array[string])=["0 -1 0\r\n", "0 -3 3 0 -3 0 -3 3 -3 0 1 0 -3 0 4 0 1 -1 0 -4 0 -3 4 -3 0 -2 2 0 -2 2 0 3 -3 0 1 0\r\n", "0 -3 0\r\n", "0 1 0 -1 0\r\n", "-1 0 3 -3 0 -3\r\n", "0 4 0 -4 0 1 0 1 0 -1 0\r\n", "-2 0 2 0\r\n", "0 -3 3 -3 0 1 0\r\n", "0 4 0 1 0 3 0 1 -4 0 4\r\n", "0 1 0 2 0 -2 3\r\n", "0 1 0 3 -3 0 -4\r\n", "0 3 0 -3 0 -4 1 0 1 0 -3 3 -3 0 -1 1 0 -3 0\r\n", "0 4 0 -1 0 3 -3 0 3 0 -3 4 -3 0 -3 3\r\n", "0 3 -3 0\r\n", "0 -1 1 0 -3 3 0 -2 2 0 2 0 3\r\n", "0 -3 3 -3 0 -3 4 -3 0 -2 2\r\n", "0 1 0\r\n", "0\r\n", "0 2 0 2 0 -3 0 4 0 1 0\r\n", "0 3 0 -2 2 0 -2 3 -3 0 -2 2 -1 0 1\r\n", "0\r\n", "-4 1 0 -1 0 3 0\r\n", "0 4 -3 0 -2\r\n", "-2 2 0 4 0 -1 0 -3 0 1 0 3 0 4 0 2 0 3 0\r\n", "0 2 0 -4 1 0 3 -3 0 2 0 3 -3 0 1 0 2 0 -3 3 -3 0 -2\r\n", "0 4\r\n", "-4 1 0 4 0 2 0\r\n", "0 1 0 3 -2 0 -3 3 0 3 -3\r\n", "0 4\r\n", "0 3 0\r\n", "0 -1 0\r\n", "0 1 0 -1 0 3 -2 0 3 -2 2 0 1 0 -3 0 4 0 2 0 -3 0 3 0 -1 0 -4 0\r\n", "-2 2 0 -3 3 -3 0 1 -4 4 -3 0 -4 1 0\r\n", "0 1 0 -2 0\r\n", "0 2 0 -2 2 0 3 -3 0 -1 0\r\n", "0 -3\r\n", "0 -1 0 -3 0 -2 3 -2 2 0 3\r\n"]
  in  "CL top vs WZ":string[](array[string])=["-4 1 0 4 0 3 0 4 0 2 0 1 -1 0 3 0 -2 2 0 -2 3 0 4\r\n", "0 -1 2 -1 0 4 -4 1 -1\r\n", "2 -1 0\r\n", "-1 0 -1 1 0 -4 4 -4 0\r\n", "0 -1 0 4 0 2\r\n", "1 0 -1 0 -1 2 0 2\r\n", "-1 0\r\n", "0 -1 1 -4 0 4 0 2 0\r\n", "0 -1\r\n", "0 2 -2 2 0 3 0\r\n", "-4 1 0 3 -2 2 -1 0 -3 0 -2 2 0\r\n", "2 0 -3 0 3 0\r\n", "0 4 0 2 0 3 0 -1 0 -2 3 0 4 -4 1 0 -1 2 -1 0 4 0 1\r\n", "-4 1 -1 0\r\n", "0 -2 0 -1 0 1 -4 1 -1 0 3 0 1 0 2 0 3 -2 0 4 0 2 0 1 0 -2 0\r\n", "0 1 0 1 0 4 0 -2\r\n", "-1 0 -1 0 2 -1 1 -1\r\n", "0 3 0 2 0 -1 1 0 4 -4 0 -1 0 -4 4 0 2 0 3\r\n", "0\r\n", "0 2 -2 2 0 -4 1 -1 0 3 0 1 0 4\r\n", "-4 1 0 1 0 4\r\n", "0 -1 0 4 0 1 0 -2 0 1 -4 4 -3 0 2\r\n", "-4 0 1 0 -1 0 4 0 4 -4 1 -1 0 3 -2 0 -1 1 0 4 0 4 -3 0 4 -4 1 -4 4 0 4 -4 0 -2\r\n", "2 0 1 0 -1 1 0 4 0 -1 0 1 -4 0 3 0 4 0 1 -4 0 -3 0 -2 3 0 -4 4 -4 0 3\r\n", "0 1 0 4 -4 0\r\n", "0 4 -4 0 -1 0\r\n", "-4 1 -1 0\r\n", "2 0 -4 0 -1 0 1 0 4 0 -1 0\r\n", "0\r\n", "0 -3 0 -1 2 0 -3 0 4 0 -2 2 0 -4 1 0 4 0 4\r\n", "-4 1 -1\r\n", "0 3\r\n", "0 -1 2 -1 0 -2 2 0\r\n", "2 0 2 0 2 -1 0 2 -2 2 0\r\n", "0\r\n"]
  in  "WZ botom vs CL":string[](array[string])=["0 3 0 -2 0 4 0 2 -2 0 4 0 4 -4 1 -4 0\r\n", "2 0 -3 3 0 -2 0 1\r\n", "0 3 0\r\n", "-4 0 2 0 3 -3 0 -3 4 0 -4 1\r\n", "-2 2 0 1 -1\r\n", "0 -1 0 4 -4 1 -4 1\r\n", "-4\r\n", "-2 2 0 3 0 -4 0 -3 3\r\n", "-4 1 0 4 -4 1 -4\r\n", "0 4 -4 0 4\r\n", "0 4 0 -4 0 1 -4 0 -4 4\r\n", "0 1 -4 0 -4 0 -2\r\n", "-2 2 0 -4 1 0 -4 0 4 0 3 0 -1 1 -1 1 0 -3 0 -2 2 0 -4 4 -4 0 2\r\n", "0 -3 3 -3 0\r\n", "-4 0 -1 2 0 -3 4 0 2 -2 0 3 -3 0 1 -4 0 -4 0 -4 0 -3 3 0 -3 4 0 2\r\n", "-2 0 3 0 -2 2 -2 0 -2 0\r\n", "-4 0 3 0 -4 1 0 -3 4\r\n", "-2 2 0 2 0 -2 0 -3 3 0 -4 1 0\r\n", "-4 0\r\n", "0 -3 3 0 2 0 -3 4 0 -2 0 1 -4 0\r\n", "0 2 0 3\r\n", "0 4 -4 1 -1 2 0 -3 0 1\r\n", "0 -2 0 -3 4 0 1 -4 0 -3 3 0 -4 0 4 0 2 -2 0 -2 0 -4\r\n", "0 3 -2 0 4 0 4 0 -1 0 -3 3 0 1 -4 0 -4 0 4 0 2 -2 0\r\n", "-2 3 -2 0 1 -4\r\n", "-4 0 -1 0 -3 3\r\n", "0 4\r\n", "0 3 0 -3 3 -3 0 -1 0 2 -2\r\n", "-2\r\n", "-4 0 -2 0 2 0 1 0 -4 0 4 0 2 0 -3 4 0 2 0 -2 0\r\n", "0 2\r\n", "-2 0\r\n", "-4 0 3 0 -4 1 -4 0 -4 4 -4 4\r\n", "0 1 -4 0 -3 3 0 1 -4 0\r\n", "-2\r\n"]
  in  "WF top vs CJ":string[](array[string])=["2 -1 0 4 0 1 0 3 -2\r\n", "0 3 0 -2 3 -2 0 -2 3 -2 2 -1 0 3 0\r\n", "1 0 1 0 4 -4 0 3 0 3 -2 0 4 0 3 -2\r\n", "0 3 -2 0 -1 1 0 2 -2 2 0 -3 4\r\n", "2 0 4\r\n", "0 -4 4 -4 0 1 -1 0 4\r\n", "-1 0 4 -4 0 -4 4 -4 0 2 0 -4 0 -3 3 -2 3 -2 0 -4\r\n", "2 0 -1 2 -1 0 1 -1 0 3 0 -2 0 3 0 -3 0 -3 0 -4 4 -4 1 -1 2 -1 1 0 3 0\r\n", "0 3\r\n", "1 0 -3 0 1 -4 0 2 0 -2 3 0 4 -4 0 -1 0 3 0 1\r\n", "0 -1 2 0 -3 4 0 -1 0 4 -4 4 -4 0 2 -1 1 0 -3 3 0\r\n", "0 3 -2 3 0 4 0 1 0 4 0 -4 4 -4 0 -4 4 -4 0 3\r\n", "2 0 3 0 1 0\r\n", "1 0 -4 1 -1 0 -2 -1 3 -2 2 -2 0 -3 0 1 -1\r\n", "2 0 3\r\n", "-4 1 -1 0 3 0 3 0 1\r\n", "0 4 0 -4 1 0 1 0 3 0 4 -4 0 -4 4 0\r\n", "2 0 -4 4 0 -1\r\n", "0 3 -2 2\r\n", "0 4 0 1 -4 4 -4 0 2 0 -3 4 0 4 -4 0 3 0 -1 1 -4 4 0 1\r\n", "0 1 -1 0 -4 0 4 0 1 0 4 0 2 0 -4 4 0 2 0 3 0 4 -4 0 3 0 4 0 -4 4\r\n", "1 0 -4 4 0 2 -1 0\r\n", "2 0 4 -4 1 -1 0 4 0 -2 2 0 4 -4 0 1 0 4 0 2\r\n", "0 4 0 3 -2 0 4\r\n", "0 3 0 -2 3 0 1 -4\r\n", "1 -4 1 0 -1 0 3 -2 2 0\r\n", "2 0 -1 0 3\r\n", "0 -1 0 2 0 -3 4 -4 0 3 0 1 -1 0 -4 4 -4 0 2 -1 1 0 3 0 4 -4 0 3 0 1 0 3 -2\r\n", "2 -1 0 3 0 4 -4 0 1 -4 1 -1 0 -4 4 0 -4 0 3 -2 0 4 -4 4 -4 0 2 -2 0 1 0 4 0 3 0 3 -2 3 -3 0 3 0 -3 0 1 -4\r\n", "1 -1 0 -2 3 -3 0 -4 0 -3 0 3 -2 0 3 -2 2\r\n", "0 4\r\n", "2 0 -2 3 0 2 -1 0 -3 0 -2 3\r\n", "1 0 3 0 3 0 -2 3 -2 0 -2 3 -2 0 3 0 1 -1 0 3 0 3 0 4 -4 0 1 -1 0 3 0 -3 0 -4 4 -4 0 3 0 -1 1 -4 1\r\n", "0 -1 2 0 3\r\n", "2 0 3 -2 0\r\n"]
  in  "CJ bottom vs WF":string[](array[string])=["0 2 -2 0 3 -3 0 -4 4\r\n", "-4 0 4 0 4 0 -4 0 -2 2 0 4\r\n", "0 -3 3 0 3 0 3 -3 0 4 -4 0 -4 0 3 -3 0\r\n", "2 0 4 0 3 -3 0 1 0\r\n", "0 4 -3 0\r\n", "-4 0 3 -2 0 1 0 -2\r\n", "0 -1 1 0 3 0 4 0 -2\r\n", "0 4 0 -3 3 0 2 0 4 -4 1 -4 0 -3 3 0 3 0 2 0\r\n", "0 4\r\n", "0 3 -3 0 -3 3 0 3 0 -3 4 0 4 -4 0 2\r\n", "-4 1 0 4 -3 0 3 0 4 -3 0 2 0 4\r\n", "-2 0 1 -4 0 4 -3 0 2 -2 0 3 0 3 0 -2 2 0 4\r\n", "0 1 0 -2 0 4 -4 0\r\n", "0 4 -3 0 -1 1 0 1 0\r\n", "0 3 -3 0\r\n", "0 2 -1 0 4 -4 0 3 0 2 -2\r\n", "-4 1 0 3 0 -3 4 0 2 -2 3 -2 2 -2 0 1\r\n", "0 3 0 -2 0 -4 0\r\n", "-2 2 0\r\n", "-4 1 0 -2 0 3 0 1 0 3 0 3 0 4 0 -2 0 -2 2 -2\r\n", "-2 0 -3 4 -3 0 2 -2 3 -2 0 -2 2 -2 0 4 -3 0 3 -3 0 1 0 3 -3 0 4 -3 0\r\n", "0 3 0 -4 0 2\r\n", "0 -4 0 -2 0 -1 1 0 3 -3 0 1 0 3 0 -2 0 3 0 4 0\r\n", "-4 0 1 0\r\n", "2 0 4 0\r\n", "0 2 0\r\n", "0 2 0\r\n", "0 3 0 1 0 3 -3 0 4 0 -2 2 0 -4 0 -1 2 0 -3 4 0 -2 0 3 0 -2 0 -1 1 0\r\n", "0 2 0 4 0 2 0 3 0 -3 0 2 0 3 0 1 -4 0 -2 0 3 0 4 -3 0 2 -2 0 -2 0 4 0 -4 0 -4 1 0 2 0 4 -4 1 -1 0 2\r\n", "0 1 -4 0 2 -1 0 3 -3 0 -4 1\r\n", "0\r\n", "0 4 -3 0 -1 2 -1 0 4 0\r\n", "0 4 0 2 0 4 0 4 0 4 -4 0 -2 2 0 3 0 2 0 2 -2 0 -2 3 -2 0 1 0 1 0 2\r\n", "0\r\n", "0 2 0 4 0 -2 0 1\r\n"]
  in  "CJ top vs MOM":string[](array[string])=["0 2 -1 0 -1 0 -4 4 -4 1 0 1 -4 1 0 -1 1 -4\r\n", "1 0 -1 0 4 -4 1 -4 1 0 4 -4 -1 0 -1\r\n", "0 -3 3 0 2 -1 0\r\n", "0 -1 2 0 -3 -4 1 0 1\r\n", "2 -1 0 -2 2 0 3 -2 0 -4 4 -4 0 4\r\n", "0 3 0 -3 0 1 0 -4 4\r\n", "0 2 -1 0 2 0 4\r\n", "0 4 -4 0 2\r\n", "0 1 0 3 0 -1 0 -4 0 1 -4 0 -4 0 3 0 -4\r\n", "-4 1 -4 1\r\n", "0 -1 0 4 -4 1 -4 1 0 3 0 3 0 -4 0 -4 0 4 -4 1\r\n", "0 1 0 1 -4 1 0\r\n", "0 2 0 -4 0 -1 2 -1 0 4 -4\r\n", "1 -4 1 0 4\r\n", "0 3 -2\r\n", "2 0 -1 0\r\n", "0 2 0 -2 0\r\n", "0 4 -4 1 -4 1 0 4 -4 1\r\n", "0 3 0 -2 2 -2 2 0 4\r\n", "-3 0 -1 0 -3\r\n", "0 1 -1 0 1 0 -4 1 0 -4 4 0 2 0 4 0 -3 3 0 4 -4 1 -4 1 0 4\r\n", "-3 0 4 0\r\n", "-4 1 0 -1 0 -1 0 -2 0\r\n", "0 3 0 -1 2 -1 0 4 -4 0 -3 0 -1 1 0 2\r\n", "0 1 0 1 -4 1 0\r\n", "0 2 -1\r\n", "1 -4 1 0 4\r\n", "0 4 0\r\n", "0 2 -1 0\r\n", "0 3 -2 0 4 0 4 -4 0 2 0\r\n"]
  in  "MOM bottom vs CJ":string[](array[string])=["0 1 0 4 0 3 0 -2 0 3 0 4 0 2 -2 0\r\n", "0 3 -2 0 4 0 -2 2 -2 0 -2 0 4 0 -2 0 2\r\n", "2 0 1 -1 0\r\n", "1 0 -3 4 -3 0 -2 0 3 0\r\n", "0 3 -2 0 4 0 -3 3 0 3 -2 0\r\n", "2 0 3 0 1 0 3\r\n", "1 0 3 -3 0 4 -3 0\r\n", "-2 2 -2 0\r\n", "0 1 0 -3 4 0 3 -2 3 0 1 0 4 0 -1\r\n", "0 3\r\n", "-2 2 0 3 0 -2 0 2 0 -2 0 3 0 -4 0 -2\r\n", "0 3 0 -3 4\r\n", "0 3 -2 2 -2 3 -2 0\r\n", "-1 0 3 0 3\r\n", "2 0\r\n", "0 -3 0 1\r\n", "1 0 4 -4 1\r\n", "-2 2 0 4 0 -2 0 -2\r\n", "1 0 4 0 1 0 -3 3\r\n", "-2 2 0 3 -2\r\n", "1 0 -3 4 -3 0 3 0 3 0 -2 0 3 -2 0 1 -4 0 3 0 -2 0 3 -3 0\r\n", "-2 2 0 2 0 3\r\n", "0 3 -2 0 3 0 -4 1\r\n", "0 1 0 -4 4 0 -2 0 3 0 -4 0 4 0 -4 1 0 3 -2 3 0 -1 1 -1\r\n", "2 0 -3 4 -3 0 2 0\r\n", "0 3\r\n", "0 3\r\n", "-1 0 4\r\n", "0 3\r\n", "-2 3 0 1 -4 0 -2 2 -2 3 0 4\r\n"]
  in  "MOM top vs CJ":string[](array[string])=["-2 2 -1 0 1 -4 0 3 -2\r\n", "1 -1 0 4 0 2 -2 3 0 1 -4 1 0 -3 4 0 3 0 4 0 4 0 -4 0\r\n", "-1 0 4 -4\r\n", "-1 0 -1 2 0 2 0\r\n", "-1 0 3 -2 0 2 -2 3 -2 2 -2 0 -3 4 0 1\r\n", "-2 2 -1 0 2 0 3 -1 3 -2 2 0 -2 2 -2 0 1 0 2 0\r\n", "1 -4 1 0 4 -4 0 2 0\r\n", "2 -2 0\r\n", "0 4 -4 -1 0 -1 1 -1 0 4 0 -2 3 -2 0\r\n", "-1 0 2 -1 0 4 -4 0 -4 0 4 0\r\n", "0 -3 0\r\n", "1 0 -1 2 -1 0 3 0 3 -2 3 -2 0 2\r\n", "2 0 2 0 -2 3 -2 2 -1 0 4 0 2\r\n", "-1 1 -4 1 0 1 0 -4 4 -4 0 3 -2 2 -1 0 3 0 -1 1\r\n", "2 0 -1 1 -1 0 3 -2 3 0 2 0 3 -2 0 -4 0 4 -4 0 4 0\r\n", "0 -1 0 3 0 2 -2\r\n", "1 -4 1 -1 0 2 0 3 -2 3 -2 3\r\n", "2 0\r\n", "-1 0 3 0 3\r\n", "1 -4 1 0 -4 4 -4 0\r\n", "-2 2 -1 0\r\n"]
  in  "CJ bottom vs MOM":string[](array[string])=["-1 0 -3 3 0 1 0 4\r\n", "0 1 0 1 0 4 0 -2 2 0 4 0 -2 0 1 0 3 0 3\r\n", "-4 1 0\r\n", "2 0 -1 0 4 -3 0 3 0 -2\r\n", "-4 0 4 0 -4 1 0 -4 0 -4 4 0 3 0\r\n", "0 3 -3 0 2 -2 0 -4 4 -4 0 -3 3 0\r\n", "0 -2 2 -2 0 3\r\n", "0 -4\r\n", "0 2 -2 0 2 0 -2\r\n", "-4 1 0 4 0 -2 2 -2 0 -2 3 -2 0 1 0 1 0 3\r\n", "0 2 0\r\n", "0 -3 3 -3 0 3 0 1 -4 0 3 0\r\n", "0 -3 4 0 1 -4\r\n", "0 3 0 -2 0 2 -1 0 2 -2 0\r\n", "0 4 -3 0 2 0 4 -3 0 -2 2 -2 0 -2 0 4\r\n", "-4 0 1\r\n", "0 -3 0 -3 0 4 0\r\n", "-1 0 1 0\r\n", "0\r\n", "0 3 0 3 -3 0 3 -3\r\n", "0 -3\r\n"]
  in  "CJ top vs HY":string[](array[string])=["0 1 -1 1 -1 1 0\r\n", "1 0\r\n", "2 -2 0 3 0 4 0 -1 0 -1\r\n", "0 4 -4 1\r\n", "0 4 -4 0 4 0 -4 1 -1 0 -3 3 0 4 -4 0 -1 0 4\r\n", "-4 0 -3 0 -4 0 2 0 4 0 -2 0 -1 1 0 4 -4\r\n", "0 -1 1 0\r\n", "0 4 0 1 -1 0\r\n", "0 2 -1 0 -4 4 -4 0 -1 1\r\n", "2 0 2 0 2 0 -3 0 4 -4 1 0\r\n", "1 0 4 0 2 0 -2 3 -2 0 4 -4 0\r\n", "0 4 0 2 0 4\r\n", "-1 1 -1 2\r\n", "0 4 -4 0 -1 2 0 -4 1 -4 4 -4 0 -4 4 -3 0 4 -4 1 0 3\r\n", "0 -1\r\n", "2 0 2 0 2\r\n", "0 3 -2 0 -1 1 -1 0 -3 0\r\n", "2 0\r\n", "0 3\r\n", "0 4 -4 1 0 3 -2 2 -2 2 0 4 0 4 0\r\n", "-4 0 -2 0 2 0 4 -4 1 -4 1 0 1\r\n", "0\r\n", "0\r\n", "0 4\r\n", "-2 2 0 -1 0 4 -4 1 0 1 -1 0 1 0 4 0 -4 4 0 2 0\r\n", "0 -1\r\n", "1 0 4 0 -2 0 -2 0 1\r\n", "2 0 -4 0 4 -3 0 1\r\n", "0 -1 1 0 -4 0\r\n", "-4 1 0 -4 0 -1 1\r\n", "0 4 0 2\r\n", "0 3 2 3\r\n", "2 0 -4 1 -4 4 -3 0 2 -1 1 -1 0 4 0 -3 0 2 0 3 -2 2 0 3\r\n", "0 1\r\n"]
  in  "HY bottom vs CJ":string[](array[string])=["-2 2 -2 0 -1\r\n", "0 4 -3 0\r\n", "0 1 0 -1 1\r\n", "-4 0\r\n", "-2 0 3 0 1 0 3 -2 0 -1 0 4 0 3 0 -3 3 -3\r\n", "0 4 0 -2 0 1 0 -4 4 -3 0 1 0 4 0 -4 1 0 3 -3 0\r\n", "0 -1 2\r\n", "2 0 -3 4 0\r\n", "-4 0 -3 3 -3 0 -3 3 0 -2 3 0\r\n", "0 -1 1 -4 4 -3 0 3 0\r\n", "0 -1 2 0 3 0 1 -4 4 0 2 0\r\n", "2 -2 0 -4 0 -4 4 0 -4\r\n", "1 -1 2 -1\r\n", "2 0 -2 0 4 0 2 0 3 0 -2 0 -4\r\n", "1 -1 0 -1\r\n", "0 1 -4 1\r\n", "0 4 0 -1 1 -1 0\r\n", "0 3\r\n", "-2 0\r\n", "1 -4 0 -2 0 4 0 -4 0 4 -3 0 1 -4 0 1\r\n", "0 -3 3 -2 0 3 0 -2 2\r\n", "1 0\r\n", "2\r\n", "0 -4\r\n", "0 4 0 -4 0 -3 3 -3 0 -2 0 -2 0 4 0 -1 1 0 3 0 -4 1 -4 0 4\r\n", "2 0 -1 1\r\n", "0 2 0 4 0 4 -4 0 -1 2\r\n", "0 3 -2 0 3 -2\r\n", "1 0 -3 3 0 -4\r\n", "0 -3 3 0 -1 0\r\n", "2 -2 0 1\r\n", "-4 1 -4 1 -4 0\r\n", "0 4 0 2 0 -4 1 2 -1 0 4 0 1 0 4 -4 4 0 -4 4 0\r\n", "-2 0 3 0 -2 0\r\n"]
  in  "HY top vs CJ":string[](array[string])=["0 4 0 4 0 4 0 4 0 -2 3 0 3 0 4 0\r\n", "-4 -1\r\n", "-2 0 1 0 -4 4\r\n", "0 4\r\n", "-2 2 0 -1 -4 1 0 3 0\r\n", "-1 0 -1 2\r\n", "0 -1 1 0 4 0 3 -2 0 -2 3 -2 0 4 0 -2 2\r\n", "2 -1 0 4\r\n", "0 4 0 2 0 -2 0\r\n", "1 -1 0 3 0 -4 4 -4 0\r\n", "2 -1 0 3 -2 0 -3 0 3 0 -3 0\r\n", "0 4 0 4 -4 1 -1 0 -3 0 1 -4 1 0 4 0 -4 0 -4 4 -4 1\r\n", "0 -4 1 0 -4 4\r\n", "0 4 0 -2 2 -2 2 -2 2\r\n", "-2 2 -1 0 4 0 2 0 4 0 2 -2 0 4\r\n", "1 0 -1 0 -1 0 1 -1\r\n", "-2 2 -2 3\r\n", "1 0 -1 0 -1 2 0 2 -2 0 -4 0\r\n", "-2 2 0 3 -2 2\r\n", "0\r\n", "1 -1 0 3\r\n", "0 4 0\r\n", "-2 0 1 -4 0 -3 0\r\n", "1 0 -1 2 -1 1 -4\r\n", "0 4\r\n", "-2 0 -1 1\r\n", "0 3 0 3 0 3 -2\r\n", "-4 0 -4 4\r\n", "0 4 0 -4 0 -4\r\n", "-2 2 0 4 -4 0 2 -2\r\n"]
  in  "CJ bottom vs HY":string[](array[string])=["2 0 3 -3 0 3 -3 0 4 0 4 0 -2 0 3\r\n", "0 -1\r\n", "0 4 0 3 0\r\n", "-4 0\r\n", "0 3 0 2 0\r\n", "0 1\r\n", "-2 0 -3 3 -2 0 3 -3 0 -4 4 0 1 0 -2 3 0 -3 4 0 1\r\n", "0 -1 2 0\r\n", "-4 0 4 -4 0 -2\r\n", "0 -1 0 4 -3 0 2 -2 3\r\n", "0 3 0 1 0 3 -3 0 1 0 1\r\n", "2 0 3 0 2 0 -3 4 0 -3 4 0 2 0 3 0 2\r\n", "0 3 0\r\n", "-4 0 2\r\n", "0 1 0 1 -4 4 -3 0 3 -3 4 0 2 -2\r\n", "0 4 0 2 -2 0\r\n", "0 4 0\r\n", "0 1 -4 4 -4 0 -3 3 0 -2 3\r\n", "0 1 -4 0 -4\r\n", "0 2 0 4\r\n", "0 -1 0 4\r\n", "-4 0 -2 3\r\n", "0 3 0 1 -4 0 -4\r\n", "0 1 -1 2\r\n", "0 3 -3 0\r\n", "0 4 0 -1 2\r\n", "-4 0 -4 4 0 4 0 -4 4\r\n", "0 3 -2 0\r\n", "0 3 -2 3 -2 2\r\n", "0 1 0 4\r\n"]
  in  "DU top vs CJ":string[](array[string])=["0 -1 0 -4 4 -4 1 -4 0\r\n", "1 -4 1 0 2 0 -3 0 2 0 -2 0 1 0 1 -4 4 -4 1 0 3 -2 0 -4 4 -4\r\n", "0 1 -4 4 -4 1\r\n", "0 3 0 -3 3 0 1 0 1 -4 4\r\n", "0 1 -4 0 1 -4\r\n", "0 3 -2 0 1 -4 1 0 2 0 4 0 4 0 -1 2 -1 0\r\n", "1 0 -1 0 2 0 4 -4\r\n", "-4\r\n", "-1 0 4\r\n", "0 1 -1 0 1 -4 0\r\n", "-1 0 1 -4 0 3 0 2 0 4 0 -4 4 -4 0 -1 0 -4 0 -2 0 4\r\n", "0 4 0\r\n", "0 4 -4 0 2 -1 0 2 0 4 -4 1 -4 4 0 3\r\n", "0 4 0 2 0\r\n", "1 0 -1 1 0 -4 1 -4 1 0 -4\r\n", "0 3 -2 0 -4\r\n", "2 -1 0 -4 4 -4 0 2 0 4\r\n", "1 0\r\n", "-1 0 -1 1 0 -4\r\n", "0 3 0\r\n", "0 -4 4 -4 0 -4 0 4 0 2 0 1 -4 4\r\n", "-1 0 1 -4\r\n", "-1 0 2 -1 0 2\r\n", "1 -1 0 4 -4 1\r\n", "-1 0 1 -4 4 -4 0 -4 4\r\n", "0 3 0 3 0 1 -1 0 1\r\n", "-1 0 4 0 4 -4 1 0 -4 0\r\n", "1 0 4\r\n", "0 -1 0 2 -1 0 -2 3 -2 0 -4 4 -4\r\n", "0 3 0\r\n", "2 -1 0 1 -4 4 -4 0 2 0\r\n", "0 4 -4 1 0 1 0 1 -4 0 2 0 4 0 4 -4 1\r\n", "1 -1 0 3 0 3 0 1 0 4\r\n", "0 -4 0 -2 0 -4\r\n", "0 -4 4 -4 0 -2 0 2 0\r\n", "-1 0 4 -4 0\r\n", "1 0 -1 2 0 4\r\n", "0 2 0 -2 0\r\n", "0 1 -4 0 -4 0 3 -2 0 -4 0 -4 4 -4 1\r\n"]
  in  "CJ bottom vs DU":string[](array[string])=["0 1 0 3 -2 3\r\n", "0 2 -2 3 -3 0 -3 3 -2 2 0 -4 4 -4 1 0 4 0 2 -2 0 4 0 4 0 2 -2 2\r\n", "0 -3 3 0 -2\r\n", "1 0 -2 0 4 0 1 0 -2 2 -2\r\n", "-2 0 3 0\r\n", "-4 0 -2 0 3 -3 0 -2 2 -2 0 -4 0 3 -2 0\r\n", "0 -3 4 0 1 0 -2\r\n", "-2\r\n", "-4 0\r\n", "-2 0 -3 4 -3 4 -4\r\n", "0 1 -4 0 -2 2 -2 0 -4 0 -3 3 -2 3 0 1 0\r\n", "0 3\r\n", "0 2 0 3 0 1 0 -2 2 -2 3 0\r\n", "-1 0 -1 1 0 4 -4 4 -4\r\n", "0 -3 4 -3 -2 2 -2 3 -2 2 -2 0\r\n", "2 0 -3 3\r\n", "0 3 0 -1 0\r\n", "0 3\r\n", "0 3 0 3\r\n", "-4 0 -4 1 -4\r\n", "2 -2 0 3 -3 0 1 0 -1 0 4 -3 0 2 -2 0\r\n", "0 1 0 4 -4 4 0\r\n", "0 1 0 -3 3 -3 0\r\n", "0 -3 4 0 -4 1 0 -2\r\n", "0 3 0 -2\r\n", "2 0 -3 3 -2 2 0 -2 0 -3 4 -3\r\n", "0 1 0 3 0\r\n", "0 3 0 -2\r\n", "-4 0 3 0 2 -1 0 3 0\r\n", "2 0 4 0 -2 2\r\n", "0 -3 4 -3 0 -2 2 -2 0 4\r\n", "0 3 -2 0 -3 4 0 3 0 1 -1 0 -1 0\r\n", "0 -3 4 -3 0\r\n", "2 0 3 -3 0 -4 0 -2\r\n", "-1 0 3 -3 0 1 0 4\r\n", "0 1 0\r\n", "0 -1 0 -1 1 -1 0\r\n", "0 -3 3 -3 0 1 -4 0 -1 0\r\n", "2 0 3 -2 0 -2 3 -2 0\r\n"]
  in  "CJ top vs DU":string[](array[string])=["0 3 0 1 0 -3 0 -3 3 0\r\n", "1 -4\r\n", "2 0 2 0 -1 0 -3\r\n", "0 4\r\n", "0 -1 2 -1 0 2 0 3 0 1 -4 1 0 -4 4 -4\r\n", "0 -1 0 -4 0 -2 0\r\n", "1 -1 1 0 -4\r\n", "-1 0 -4 0 1 0\r\n", "0 3\r\n", "-1 1 0 -4 1 0 -4 0 -1 2 0\r\n", "1 0 -1 0 2\r\n", "0 -1 -4 1 0 -3 3\r\n", "2 -1 0\r\n", "0 4 0 2 0 -3 0 1 -1 0 1 -4 4 -4 4 -4 0 3\r\n", "0 -4 4 -4 0 -1 2 0 3 -3 0 -3 3 0 -4 1 0 -3 0 3 -2\r\n", "0 3 0\r\n", "0 4 0 1 0 -4 4\r\n", "0 -1 0 4 0\r\n", "1 -1 0 4 0 2 -2 0 -4 1 -4 4 -3 0 -4 0 -3 3 0 -4 1 -1 2 -1 0 4\r\n", "0 3 0 4 -4 4 -4 1 -4 1 -4 4 -4 1 -4 0 -3 3\r\n", "", "0\r\n", "0 4 -4 0 -4 0 4 -4 0\r\n", "1 -4\r\n", "0 4\r\n", "0 1 -4 1 -4 0 -4 4 -4 0\r\n", "-2 2 0 -3 3 -3 0 3 0\r\n", "1 0 4 0\r\n", "0 3 0 1 0\r\n", "0 4 -4 0 -4 1 -4 0\r\n", "0\r\n", "0 -4 4 -4 0 -3 3 -2 0 2\r\n", "0 3 0 1 0 -4 4 0 -3 3 0 -4 0\r\n"]
  in  "Du bottom vs CJ":string[](array[string])=["-2 0 3 0 -3 0 4 -4 0\r\n", "0 3\r\n", "0 4 -3 0 -4 1 0 4 -3 0\r\n", "0\r\n", "-2 0 3 -3 0 -4 1 -4 0 3 -3 4 -3 0 2 0 3\r\n", "0 3 0 1\r\n", "0 1 0 3\r\n", "0 3 -2 0 4\r\n", "0\r\n", "0 -3 4 0 2 -2 0 -3 0 3 -2 3 -3 4\r\n", "0 -3 4 -3 0\r\n", "-2 0 -2 2 0\r\n", "0 3 -2\r\n", "0 4 -3 0 3 -2 0 -3 4 -3 0 3 -2 2 -2 0 4 0\r\n", "2 0 1 -4 0 3 0 -4 4 0 -4 4 0 2 0 4 0 -3 4 -3 0 -4 0 4\r\n", "0 4\r\n", "-2 0 -2 0 3 0\r\n", "0 3 0 -2 3\r\n", "0 4 0 4 -4 0 2 0 -4 4 -3 0 -2 2 -2 0 4 -3 0 2 0 3 0\r\n", "0 4 -3 0 1 -1 0 3 0 -2 2 -2 0 -3 4 -3 0 4 -4 1 0\r\n", "", "0 -3\r\n", "2 0 3 0 1 0 -2 3\r\n", "0\r\n", "1 -1 0\r\n", "0 -2 3 0\r\n", "0 1 0 4 0 4 -4 4\r\n", "0 1 -1 0 3\r\n", "0 2 -2 3 -3 4\r\n", "-2 2 0 -2 3\r\n", "0 -1\r\n", "0 4 -4 4 0 3 0 -2 0 -4 0 1 -4\r\n", "-2 0 4 0 -3 3 0 -2 2 -2 0 -4 0 4 0\r\n"]
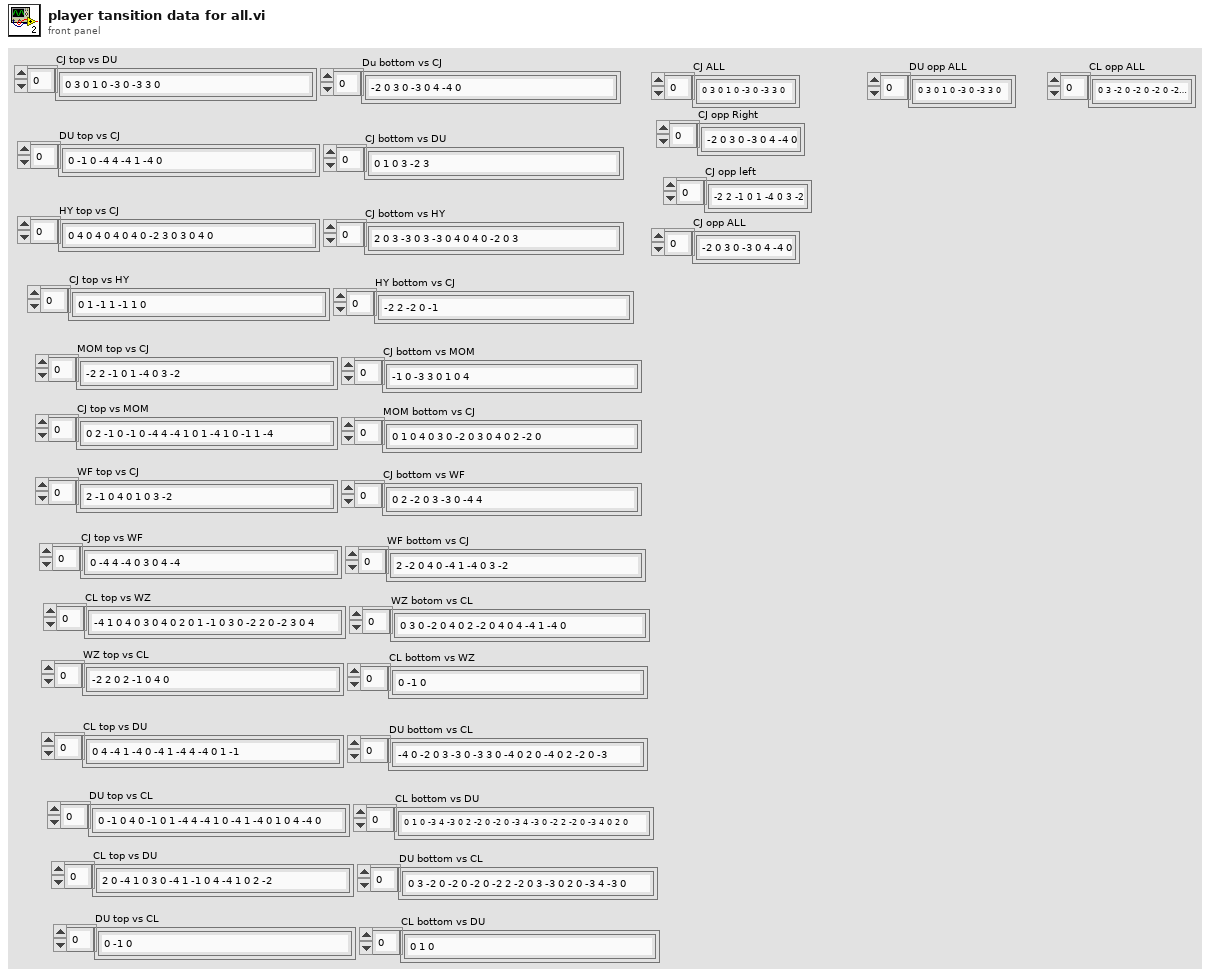
[diagram p1: front panel]
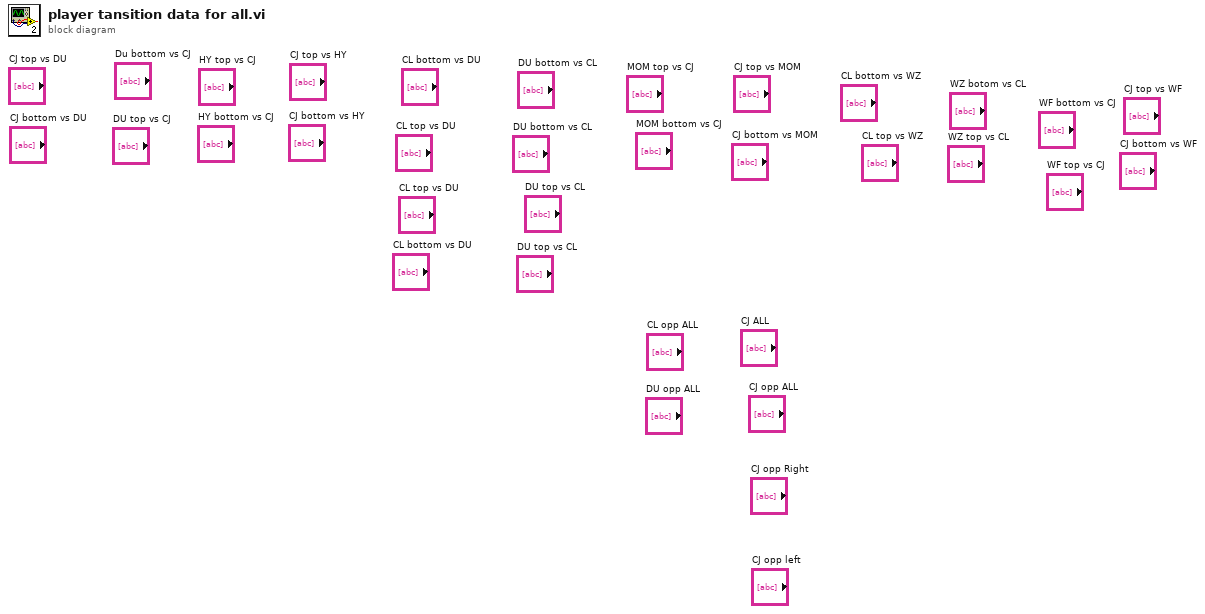
[diagram p0: block diagram]
diagram:
